vi "diSPIM Control_dual color_AB_v8.vi"(1 "Prefix for image filenames":string="A549-R11AGFP-RFP-RSV-mock-7", 3 "File Path to save DCIMG files":path=path "E:/DATA/20180315/mock") -> ()   [LabVIEW 2016]
uses:
  <userlib>/Lumenera/NiLuApi.lvlibp/Controls/LuProp.ctl
  <vilib>/DAQmx/write.llb/DAQmx Write (Analog 1D Wfm NChan NSamp).vi
  <vilib>/DAQmx/create/channels.llb/DAQmx Create Channel (AO-Voltage-Basic).vi
  <vilib>/DAQmx/configure/timing.llb/DAQmx Timing (Use Waveform).vi
  <vilib>/DAQmx/miscellaneous.llb/DAQmx Fill In Error Info.vi
  <vilib>/Instr/_visa.llb/VISA Configure Serial Port (Instr).vi
  <vilib>/ErrorRing/Error Ring.xnode
  <resource>/objmgr/daqmx.rc
  <vilib>/measure/NI_MABase.lvlib
  <userlib>/Lumenera/NiLuApi.lvlibp
  <vilib>/vision/NI_Vision_Development_Module.lvlib
panel:
  in  "Control Mode:":T1(ring) caption="Enum"
  in  "Tab Control":T2(tab)
  in  "Tab Control 4":T3(tab)=enum."SPIM Head Control"
  in  "Piezo Conversion Factor (V)":dbl=0.066
  in  "Z-Galvo Conversion \nFactor B (V)":dbl=0.0065
  in  "Z-Galvo Conversion \nFactor A (V)":dbl=0.0066
  in  "Imaging Piezo Offset (V)\n(SPIM ARM B)":dbl=5.149 min=0.0 max=10.0 step=0.001 format="%_4g"
  in  "Y-Galvo Offset B (V)":dbl=2.5 min=0.0 max=5.0 step=0.001
  in  "Imaging Piezo Offset (V)\n(SPIM ARM A)":dbl=5.487000000000003 min=0.0 max=10.0 step=0.001 format="%_4g"
  in  "Y-Galvo Offset A (V)":dbl=2.5 min=0.0 max=5.0 step=0.001
  in  "Z-Galvo Offset B (V)":dbl=2.5139999999999985 min=0.0 max=5.0 step=0.001 format="%_4g"
  in  "Z-Galvo Offset A (V)":dbl=2.5239999999999894 min=0.0 max=5.0 step=0.001 format="%_4g"
  in  "lower by":dbl=1.0 caption="um"
  in  "raise by":dbl=25000.0 caption="um"
  in  "Lower head  to 1 mm":bool caption="Lower SPIM head to find cells"
  in  "Raise head to 25 mm":bool
  in  "Lower button":bool=TRUE
  in  "Raise button":bool
  in  "Halt":bool=TRUE
  in  "Tab Control 3":T4(tab)
  out "Camera 2 Details":T5={"Model"="C11440-22C", "Camera ID"="S/N: 100720", "Firmware"="4.00.A"}
  in  "Stop SPIM \nlive":bool
  out "Camera 1 Details":T5={"Model"="C11440-22C", "Camera ID"="S/N: 100719", "Firmware"="4.00.A"}
  in  "Laser beam reference":u16(ring) items=["Right Camera", "Left Camera"]
  in  "Start SPIM \nlive":bool
  in  "Imaging":bool
  in  "Epi":bool caption="beam"
  in  "Epi scanning":bool=TRUE caption="scan"
  in  "Imaging \nscanning":bool=TRUE
  in  "BottomCam \nStop button":bool
  in  "BottomCam\n Live button":bool=TRUE
  in  "Gain":sgl(slide)=13.93722 min=0 max=14 step=0.5 scale=0.0..14.0
  in  "Exposure time (ms)":sgl(slide)=223.31839 caption="ms" min=0 max=300 step=20 scale=0.0..300.0
  in  "Raise obj \nbool":bool
  in  "Lower obj \nbool":bool
  in  "Raise obj by":dbl=10.0 caption="um"
  in  "Lower obj by":dbl=10.0 caption="um"
  in  "Tab Control 2":enum32{"Cofus alignment", "Overlay parameters"}(tab)=enum."Overlay parameters"
  in  "Z-galvo Offset A slider":dbl(slide) scale=-30.0..30.0
  in  "Z-galvo Offset B slider":dbl(slide)=0.15873015873015817 scale=-30.0..30.0
  in  "Overlay Color":u32(colorbox)
  in  "Choose Overlay":u16(ring)=2 items=["No overlay", "x", "+"]
  in  "lower threshold":u16(slide)=88 scale=0.0..150.0
  in  "higher threshold":u16(slide)=20000 min=124 scale=100.0..20000.0
  in  "mid-level":u16(slide)=1709 min=124 max=50994 scale=100.0..6000.0
  out "Right spim Camera image":T6(plugin-control) caption="Right SPIM Cam"
  in  "Stop Adjustment":bool
  out "Waveform Graph":sgl[](graph)=[101.0, 104.0, 103.0, 99.0, 104.0, 97.0, 103.0, 98.0, 108.0, 97.0, 100.0, 98.0, 98.0, 99.0, 99.0, 105.0, 101.0, 103.0, 101.0, 106.0, 101.0, 104.0, 101.0, 104.0, 106.0, 87.0, 96.0, 98.0, 100.0, 99.0, 100.0, 99.0, 106.0, 103.0, 104.0, 103.0, 110.0, 104.0, 98.0, 101.0, 105.0, 100.0, 94.0, 103.0, 101.0, 105.0, 103.0, 107.0, 104.0, 103.0, 96.0, 110.0, 104.0, 99.0, 109.0, 101.0, 97.0, 98.0, 101.0, 101.0, 102.0, 107.0, 98.0, 106.0, 105.0, 108.0, 91.0, 106.0, 100.0, 101.0, 104.0, 101.0, 121.0, 105.0, 107.0, 101.0, 107.0, 101.0, 85.0, 104.0, 100.0, 104.0, 105.0, 107.0, 101.0, 103.0, 101.0, 101.0, 96.0, 107.0, 100.0, 98.0, 104.0, 101.0, 100.0, 105.0, 108.0, 104.0, 90.0, 104.0, 105.0, 103.0, 109.0, 108.0, 98.0, 105.0, 105.0, 108.0, 100.0, 109.0, 103.0, 104.0, 107.0, 103.0, 98.0, 99.0, 106.0, 106.0, 99.0, 107.0, 99.0, 100.0, 102.0, 101.0, 108.0, 98.0, 98.0, 105.0, 100.0, 100.0, 107.0, 107.0, 98.0, 106.0, 104.0, 102.0, 116.0, 108.0, 104.0, 100.0, 99.0, 100.0, 101.0, 100.0, 103.0, 108.0, 102.0, 113.0, 108.0, 110.0, 122.0, 108.0, 101.0, 110.0, 105.0, 108.0, 101.0, 107.0, 109.0, 108.0, 104.0, 114.0, 107.0, 108.0, 111.0, 102.0, 118.0, 107.0, 117.0, 117.0, 103.0, 101.0, 105.0, 110.0, 105.0, 112.0, 112.0, 115.0, 106.0, 119.0, 105.0, 115.0, 113.0, 121.0, 110.0, 108.0, 110.0, 115.0, 112.0, 113.0, 112.0, 108.0, 115.0, 109.0, 102.0, 115.0, 112.0, 113.0, 115.0, 126.0, 125.0, 105.0, 120.0, 116.0, 125.0, 122.0, 115.0, 107.0, 111.0, 136.0, 115.0, 123.0, 116.0, 126.0, 115.0, 123.0, 132.0, 142.0, 129.0, 146.0, 134.0, 145.0, 140.0, 152.0, 143.0, 148.0, 143.0, 140.0, 170.0, 170.0, 202.0, 208.0, 209.0, 234.0, 232.0, 276.0, 293.0, 298.0, 361.0, 427.0, 415.0, 450.0, 477.0, 544.0, 541.0, 653.0, 643.0, 756.0, 771.0, 801.0, 810.0, 930.0, 954.0, 970.0, 1079.0, 1072.0, 1191.0, 1148.0, 1110.0, 1097.0, 1055.0, 942.0, 881.0, 839.0, 731.0, 669.0, 626.0, 534.0, 535.0, 474.0, 363.0, 352.0, 342.0, 280.0, 315.0, 253.0, 270.0, 247.0, 229.0, 206.0, 203.0, 187.0, 158.0, 163.0, 175.0, 145.0, 154.0, 158.0, 147.0, 138.0, 121.0, 130.0, 126.0, 120.0, 131.0, 121.0, 119.0, 113.0, 120.0, 125.0, 113.0, 122.0, 130.0, 129.0, 114.0, 115.0, 106.0, 127.0, 124.0, 112.0, 120.0, 105.0, 117.0, 115.0, 125.0, 110.0, 111.0, 113.0, 124.0, 106.0, 117.0, 117.0, 119.0, 127.0, 131.0, 118.0, 124.0, 128.0, 121.0, 116.0, 108.0, 107.0, 102.0, 115.0, 112.0, 124.0, 112.0, 124.0, 108.0, 118.0, 105.0, 119.0, 109.0, 111.0, 109.0, 119.0, 108.0, 111.0, 107.0, 117.0, 111.0, 104.0, 106.0, 114.0, 110.0, 115.0, 113.0, 105.0, 118.0, 116.0, 110.0, 104.0, 106.0, 120.0, 101.0, 104.0, 102.0, 110.0, 99.0, 112.0, 112.0, 99.0, 110.0, 109.0, 115.0, 104.0, 107.0, 104.0, 108.0, 102.0, 106.0, 112.0, 106.0, 108.0, 104.0, 110.0, 108.0, 104.0, 106.0, 106.0, 96.0, 113.0, 108.0, 99.0, 112.0, 110.0, 109.0, 112.0, 107.0, 94.0, 108.0, 103.0, 106.0, 108.0, 108.0, 101.0, 113.0, 101.0, 100.0, 101.0, 107.0, 93.0, 104.0, 100.0, 100.0, 103.0, 101.0, 108.0, 113.0, 108.0, 89.0, 107.0, 105.0, 109.0, 106.0, 103.0, 106.0, 117.0, 100.0, 108.0, 103.0, 105.0, 104.0, 101.0, 100.0, 105.0, 109.0, 108.0, 105.0, 109.0, 106.0, 104.0, 98.0, 102.0, 98.0, 104.0, 107.0, 100.0, 106.0, 102.0, 101.0, 99.0, 106.0, 109.0, 101.0, 105.0, 106.0, 116.0, 101.0, 104.0, 105.0, 102.0, 106.0, 103.0, 100.0, 101.0, 101.0, 105.0, 103.0, 105.0, 108.0, 109.0, 97.0, 108.0, 105.0, 99.0, 110.0, 110.0, 108.0, 102.0, 100.0, 103.0, 109.0, 111.0, 104.0, 106.0, 108.0, 105.0, 101.0, 98.0, 100.0, 98.0, 101.0, 98.0, 101.0, 107.0, 100.0, 101.0, 101.0, 103.0, 101.0, 106.0, 101.0, 101.0, 104.0, 112.0, 101.0, 99.0, 105.0, 104.0, 100.0, 110.0]
  out "Left spim Camera image":T6(plugin-control) caption="Left SPIM Cam"
  in  "LED power":i32(slide) min=0 max=100 step=1 scale=0.0..100.0
  in  "Switch to internal":bool
  out "Scanner/Piezo \ncontrol mode":string="Already in external (NI-DAQ)"
  out "Waveform Graph 2":sgl[](graph)=[102.0, 99.0, 106.0, 109.0, 108.0, 102.0, 107.0, 106.0, 103.0, 111.0, 105.0, 99.0, 105.0, 102.0, 104.0, 102.0, 103.0, 104.0, 107.0, 107.0, 104.0, 110.0, 105.0, 106.0, 109.0, 101.0, 109.0, 101.0, 103.0, 105.0, 103.0, 101.0, 100.0, 106.0, 106.0, 100.0, 101.0, 101.0, 107.0, 101.0, 104.0, 103.0, 101.0, 111.0, 102.0, 107.0, 100.0, 104.0, 109.0, 108.0, 107.0, 101.0, 108.0, 103.0, 105.0, 102.0, 107.0, 107.0, 100.0, 98.0, 104.0, 114.0, 98.0, 106.0, 102.0, 115.0, 109.0, 111.0, 102.0, 99.0, 110.0, 116.0, 101.0, 107.0, 104.0, 106.0, 112.0, 104.0, 106.0, 95.0, 104.0, 103.0, 110.0, 107.0, 104.0, 105.0, 102.0, 110.0, 101.0, 107.0, 104.0, 111.0, 100.0, 102.0, 115.0, 111.0, 118.0, 99.0, 108.0, 100.0, 100.0, 105.0, 107.0, 105.0, 117.0, 101.0, 114.0, 112.0, 102.0, 111.0, 103.0, 113.0, 106.0, 107.0, 110.0, 105.0, 108.0, 111.0, 101.0, 108.0, 113.0, 111.0, 103.0, 112.0, 105.0, 101.0, 117.0, 111.0, 105.0, 107.0, 105.0, 114.0, 113.0, 98.0, 102.0, 115.0, 114.0, 107.0, 105.0, 113.0, 114.0, 114.0, 119.0, 111.0, 100.0, 114.0, 114.0, 106.0, 110.0, 115.0, 111.0, 108.0, 124.0, 112.0, 105.0, 123.0, 111.0, 109.0, 117.0, 111.0, 110.0, 118.0, 109.0, 111.0, 103.0, 113.0, 113.0, 111.0, 104.0, 108.0, 106.0, 123.0, 114.0, 108.0, 119.0, 118.0, 120.0, 126.0, 124.0, 108.0, 121.0, 123.0, 111.0, 122.0, 121.0, 117.0, 115.0, 126.0, 113.0, 127.0, 139.0, 125.0, 122.0, 126.0, 132.0, 162.0, 146.0, 141.0, 142.0, 130.0, 159.0, 159.0, 198.0, 172.0, 207.0, 211.0, 256.0, 274.0, 308.0, 402.0, 428.0, 376.0, 428.0, 645.0, 602.0, 716.0, 602.0, 661.0, 566.0, 594.0, 553.0, 512.0, 490.0, 361.0, 363.0, 257.0, 258.0, 264.0, 251.0, 258.0, 256.0, 262.0, 248.0, 299.0, 221.0, 221.0, 170.0, 167.0, 172.0, 150.0, 143.0, 153.0, 142.0, 156.0, 155.0, 118.0, 159.0, 150.0, 143.0, 154.0, 134.0, 144.0, 152.0, 151.0, 161.0, 169.0, 163.0, 147.0, 179.0, 176.0, 174.0, 161.0, 175.0, 217.0, 228.0, 253.0, 288.0, 374.0, 510.0, 661.0, 735.0, 851.0, 1145.0, 1247.0, 1085.0, 773.0, 617.0, 484.0, 393.0, 392.0, 316.0, 287.0, 216.0, 197.0, 195.0, 173.0, 170.0, 159.0, 147.0, 152.0, 124.0, 131.0, 116.0, 119.0, 107.0, 107.0, 113.0, 104.0, 113.0, 114.0, 108.0, 114.0, 103.0, 107.0, 105.0, 111.0, 104.0, 100.0, 101.0, 104.0, 105.0, 97.0, 98.0, 95.0, 111.0, 101.0, 108.0, 105.0, 103.0, 107.0, 114.0, 103.0, 109.0, 106.0, 107.0, 93.0, 99.0, 101.0, 104.0, 103.0, 101.0, 107.0, 100.0, 96.0, 99.0, 100.0, 104.0, 106.0, 101.0, 110.0, 108.0, 102.0, 100.0, 101.0, 105.0, 98.0, 102.0, 103.0, 101.0, 97.0, 105.0, 104.0, 102.0, 100.0, 101.0, 105.0, 100.0, 107.0, 101.0, 105.0, 101.0, 100.0, 102.0, 99.0, 103.0, 111.0, 103.0, 105.0, 102.0, 100.0, 108.0, 98.0, 101.0, 105.0, 97.0, 101.0, 100.0, 101.0, 103.0, 109.0, 103.0, 101.0, 100.0, 105.0, 99.0, 102.0, 103.0, 97.0, 107.0, 105.0, 101.0, 100.0, 101.0, 101.0, 103.0, 101.0, 101.0, 105.0, 104.0, 101.0, 96.0, 101.0, 97.0, 102.0, 103.0, 102.0, 101.0, 111.0, 103.0, 102.0, 101.0, 106.0, 100.0, 108.0, 101.0, 103.0, 102.0, 102.0, 103.0, 104.0, 100.0, 109.0, 105.0, 101.0, 100.0, 99.0, 102.0, 95.0, 98.0, 107.0, 98.0, 103.0, 104.0, 101.0, 101.0, 106.0, 101.0, 102.0, 103.0, 99.0, 103.0, 99.0, 97.0, 99.0, 100.0, 101.0, 111.0, 102.0, 100.0, 104.0, 98.0, 100.0, 118.0, 100.0, 100.0, 105.0, 100.0, 99.0, 103.0, 117.0, 101.0, 104.0, 102.0, 101.0, 100.0, 102.0, 101.0, 102.0, 100.0, 102.0, 100.0, 103.0, 99.0, 100.0, 106.0, 103.0, 102.0, 104.0, 105.0, 103.0, 99.0, 103.0, 102.0, 100.0, 99.0, 94.0, 101.0, 102.0, 101.0, 100.0, 101.0, 104.0, 106.0, 99.0, 106.0, 95.0, 100.0, 102.0, 102.0, 101.0, 101.0, 100.0, 101.0, 105.0, 95.0, 88.0, 98.0, 98.0, 100.0, 98.0, 98.0, 108.0]
  in  "Bgndbool":bool=TRUE
  in  "Autofocus \n(move only galvo )":bool
  in  "Time/Plane":dbl=5.0 caption="ms"
  in  "Z Step Size":dbl=0.5 caption="um" min=0.0 max=2.0
  in  "# Planes/Volume":dbl=50.0
  in  "# of Volumes":dbl=500.0
  in  "Time Point Delay":dbl caption="ms"
  in  "Laser power (488 nm)":dbl(slide) min=0.0 max=10.0 step=0.1 scale=0.0..10.0
  in  "Laser power (561 nm)":dbl(slide) min=0.0 max=10.0 step=0.1 scale=0.0..10.0
  in  "Light Sheet Width":dbl=40.0 caption="um"
  out "Volume Indicator":dbl(slide)=499.0 max=10.0 scale=0.0..500.0
  out "planes acquired (B)":dbl=49.0 caption="SPIM B"
  out "planes acquired (A)":dbl=49.0 caption="SPIM A"
  in  "Export to TIFF":bool
  out "Acquisition status:":string="Done."
  out "Camera A ID:":string="S/N: 100719"
  out "Camera B ID:":string="S/N: 100720"
  in  "Camera SPIMB":T7={"Horizontal Offset"=772, "Vertical Offset"=772, "Horizontal Width"=512, "Vertical Width"=512}
  in  "Camera SPIMA":T7={"Horizontal Offset"=772, "Vertical Offset"=772, "Horizontal Width"=512, "Vertical Width"=512}
  out "TIFF storage for SPIM ARM B":path=path "E:/DATA/20180315/mock/A549-R11AGFP-RFP-RSV-mock-7/ARM2"
  out "TIFF storage for SPIM ARM A":path=path "E:/DATA/20180315/mock/A549-R11AGFP-RFP-RSV-mock-7/ARM1"
  in  "AutoFocus \n(move only piezo)":bool caption="AutoFocus"
  out "SPIM Camera Error":errorcluster {"code" format="%.0x"}
  out "SPIMA DAQ Error":errorcluster
  out "SPIMB DAQ Error":errorcluster
  out "Bottom Cam error":errorcluster
  in  "X-Position":dbl
  in  "Y-Position":dbl
  in  "F-Axis Position":dbl
  in  "File Name":string
  out "DAQ1 error (adjustment)":errorcluster
  out "DAQ2 error (adjustment)":errorcluster
  out "File conversion error":errorcluster
  out "stage2":u32=267
  out "stage1":u32=268
  out "stage 3":u32=37
  out "interstage":u32=1
  out "stage0":u32=113
  out "Serial port errors":errorcluster
  in  "Capture Images On/Off":bool=TRUE
  out "stage0 2":u32=174
  out "interstage 2":u32=1
  out "stage 4":u32=54
  out "stage2 2":u32=600
  out "stage1 2":u32=547
  out "File conversion Dual color":errorcluster
  out "BottomCam\n frameRate out":sgl=20.58668
  in  "Force Cameras Open":bool
  out "Imag. cond. error out":errorcluster
  # "Galvo & Piezo Control"
  # "SPIM A"
  # "SPIM B"
  # "SPIM head motion"
  # "Scouting camera control"
  # "Storage for DCIMG image files"
  # "Image Acquisition Parameters"
  # "Imaging progress indicators"
  # "Storage for TIFF files post export"
  # "Camera Control parameters"
  # "Saving Front Panel Parameters"
  # "Single color timing"
  # "Dual color timing"
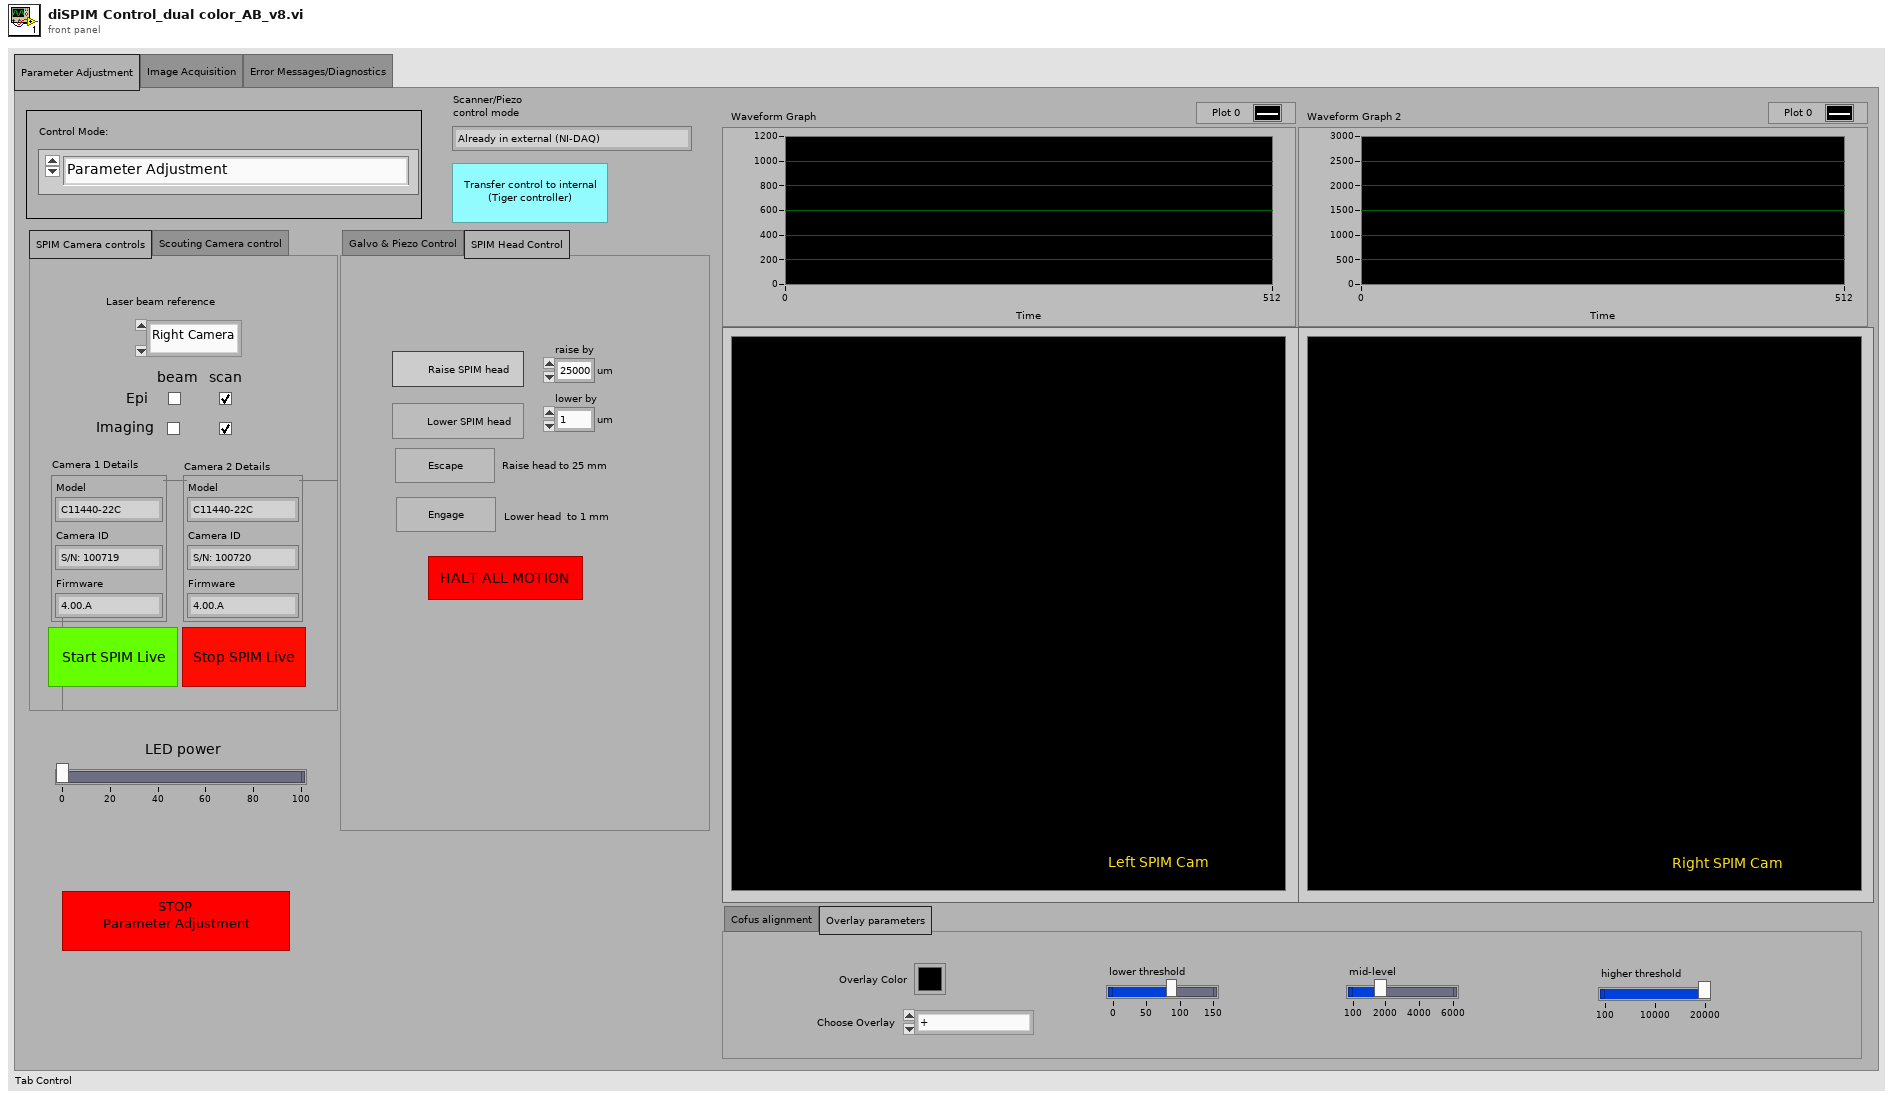
[diagram p1: front panel]
types:
  T1 = enum32{"Parameter Adjustment", "Image Acquisition - Single Color", "Image Acquisition - Dual Color"}
  T2 = enum32{"Parameter Adjustment", "Image Acquisition", "Error Messages/Diagnostics"}
  T3 = enum32{"Galvo & Piezo Control", "SPIM Head Control"}
  T4 = enum32{"SPIM Camera controls", "Scouting Camera control"}
  T5 = cluster{"Model":string, "Camera ID":string, "Firmware":string}
  T6 = typedef "IMAQ Image.ctl" = refnum<image>
  T7 = cluster{"Horizontal Offset":i32, "Vertical Offset":i32, "Horizontal Width":i32, "Vertical Width":i32}
  T8 = cluster{"cTime/plane":dbl, "cNoOfVol":dbl, "cZStepSize":dbl, "cTimePointDelay":dbl, "cPlanes/Vol":dbl, "cLightShtWdth":dbl, "cLasPow488":dbl, "cLasPow561":dbl, "cZGalOffA":dbl, "cZGalOffB":dbl, "cZGalConvFacA":dbl, "cZGalConvFacB":dbl, "cYGalOffA":dbl, "cYGalOffB":dbl, "cPzOffB":dbl, "cPzOffA":dbl, "cPzConvFac":dbl}
  T9 = cluster{"Y-Gal ampl":dbl, "A Z-Gal amp":dbl, "A Z-Gal Off":dbl, "Imag Obj Amp":dbl, "A Obj Off H":dbl, "A Obj Off L":dbl, "B Obj Off H":dbl, "B Obj Off L":dbl, "B Z-Gal Amp":dbl, "B Z-Gal Off":dbl, "488 laser pow":dbl, "561 laser pow":dbl, "A Y-Gal Off":dbl, "B Y-Gal Off ":dbl, "planes/vol":dbl, "Time/plane":dbl}
  T10 = cluster{"Demosaicing Method":u32, "Correction Matrix":u32}
  T11 = enum16{"Sine Wave", "Triangle Wave", "Square Wave", "Sawtooth Wave"}
  T12 = cluster{"height":u32, "width":u32, "datatype":u32}
  T13 = typedef "Image Type" = u32
  T14 = typedef "NiLuApi.lvlibp/LuProp.ctl" = u32
  T15 = cluster{"Size":u32, "Width":u32, "Height":u32, "Pixel Format":u32, "Image Size":u32, "Reserve 1":u32, "Reserve 2":u32, "Reserve 3":u32, "Reserve 4":u32, "Reserve 5":u32, "Reserve 6":u32, "Reserve 7":u32, "Reserve 8":u32}
  T16 = typedef "NiLuApi.lvlibp/IMAQ Image.ctl" = refnum<image>
  T17 = cluster{"DAQ1":waveform(dbl)[], "DAQ 2":waveform(dbl)[]}
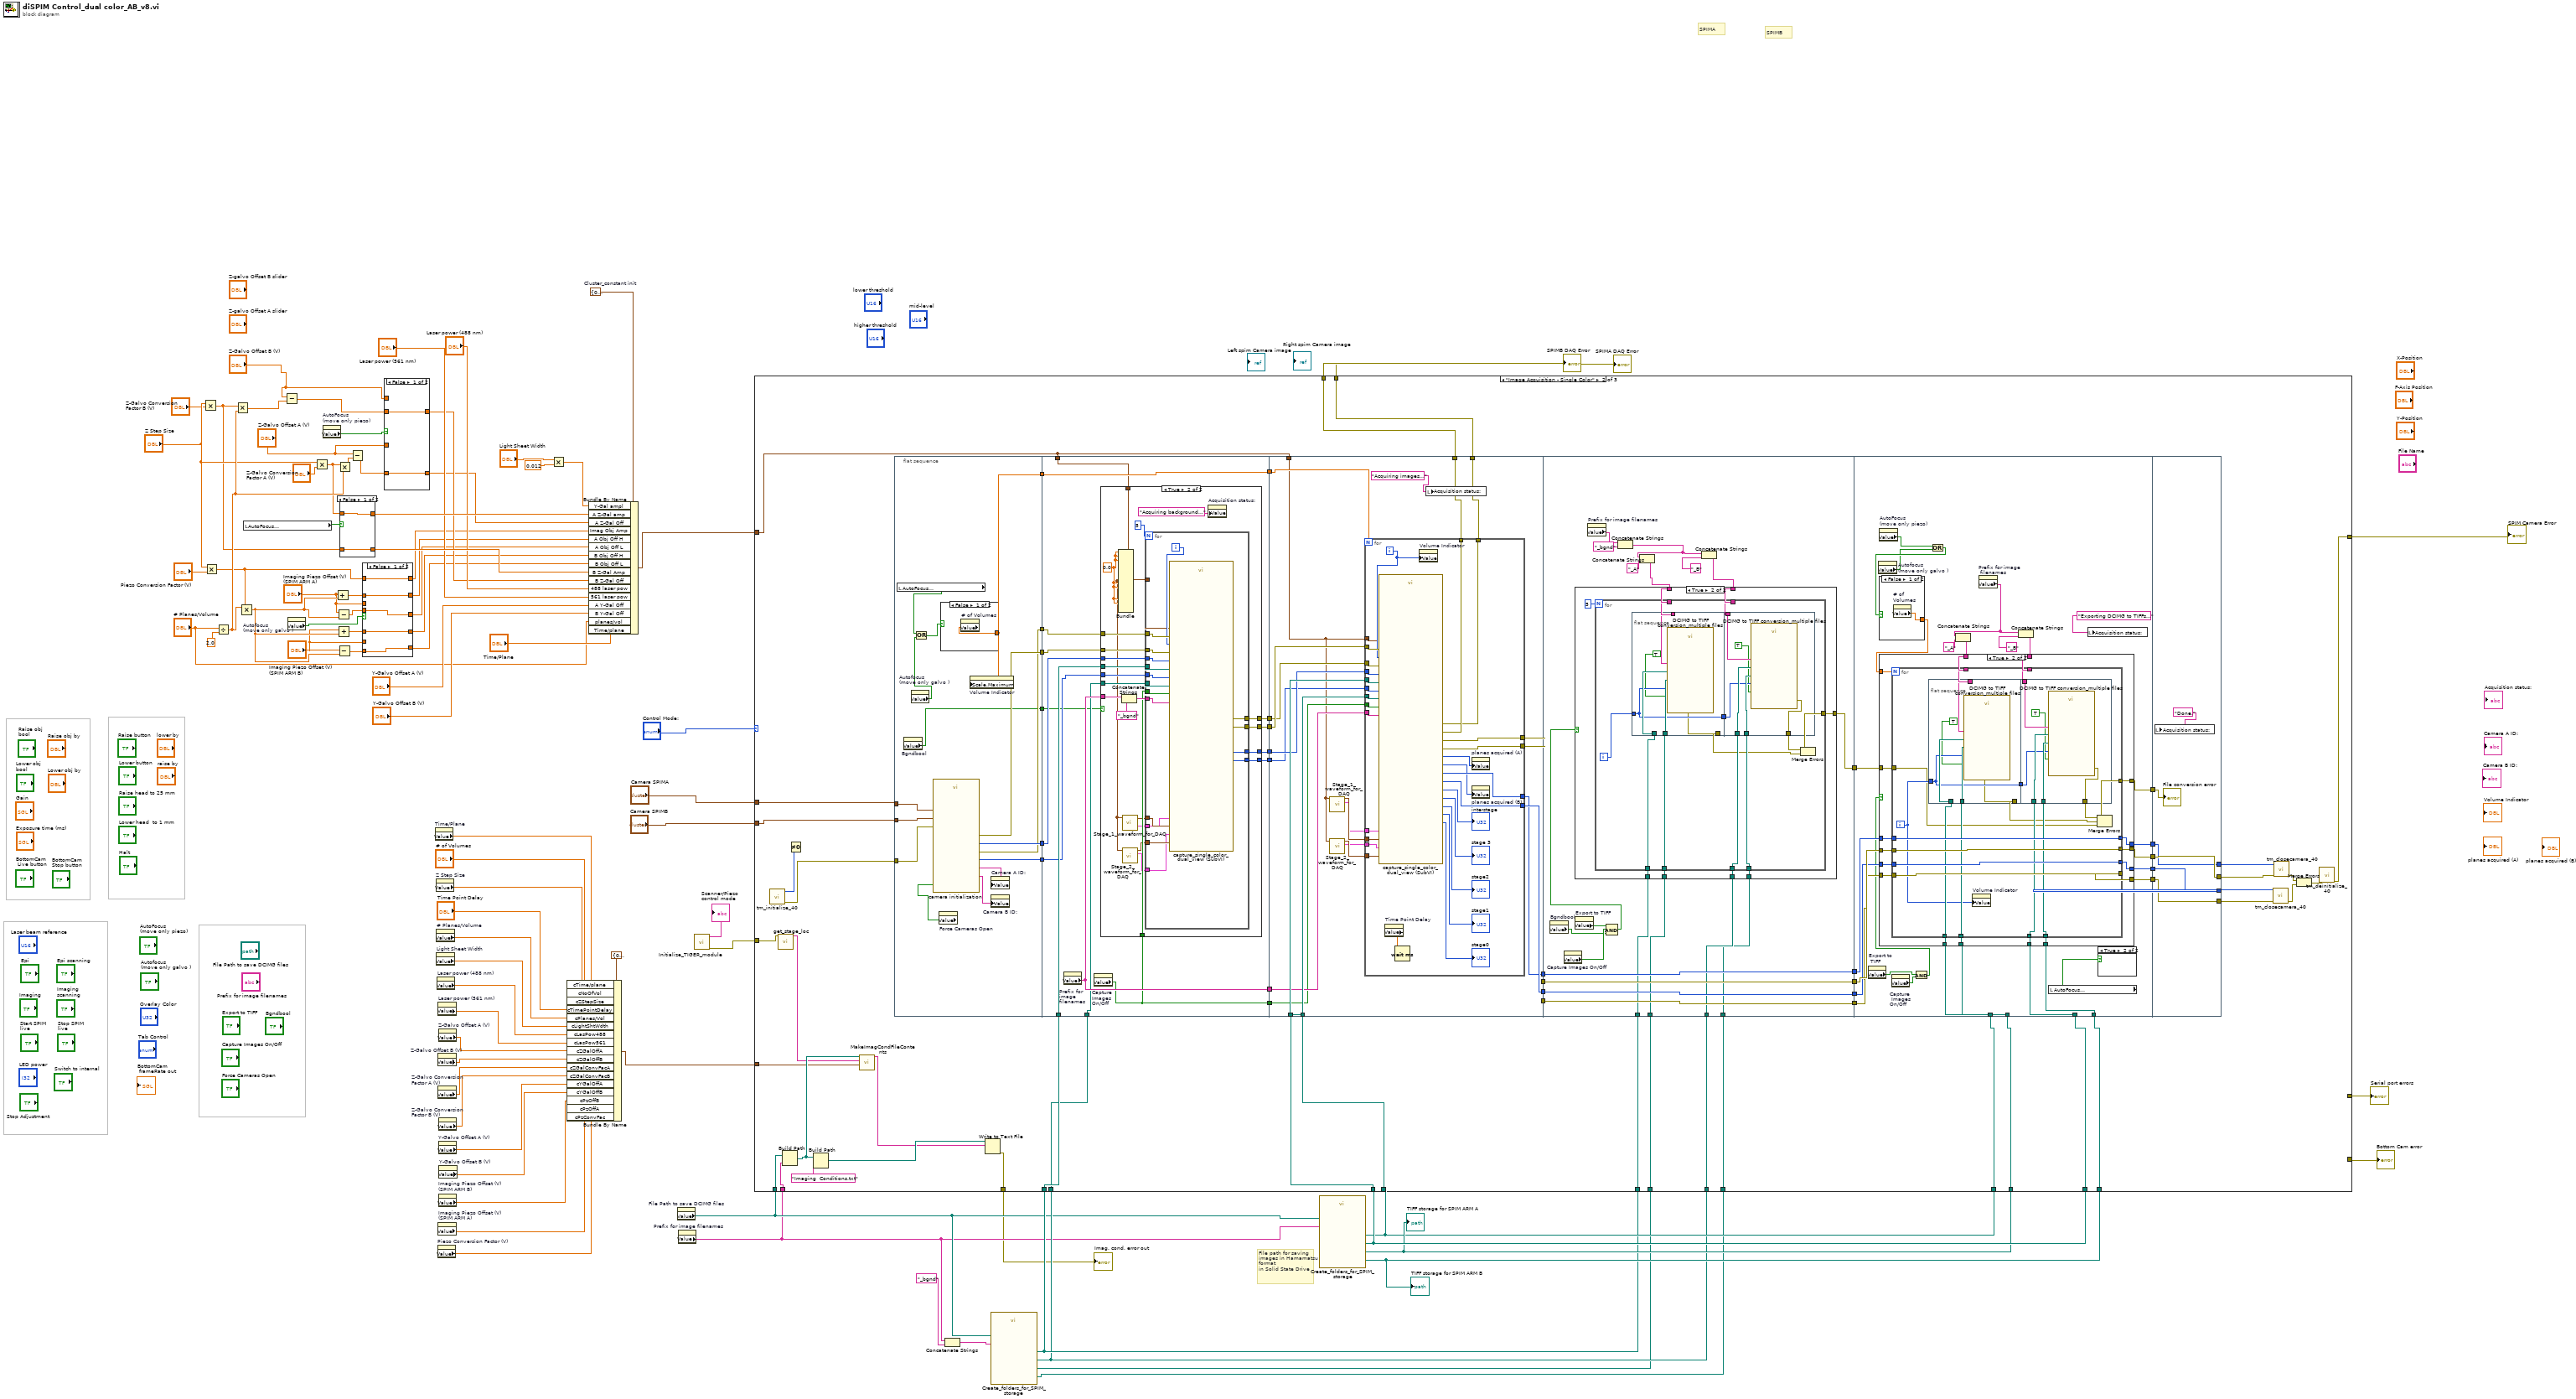
[diagram p0: block diagram]
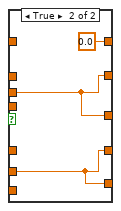
[diagram p2: hidden frame]
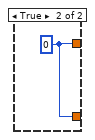
[diagram p4: hidden frame]
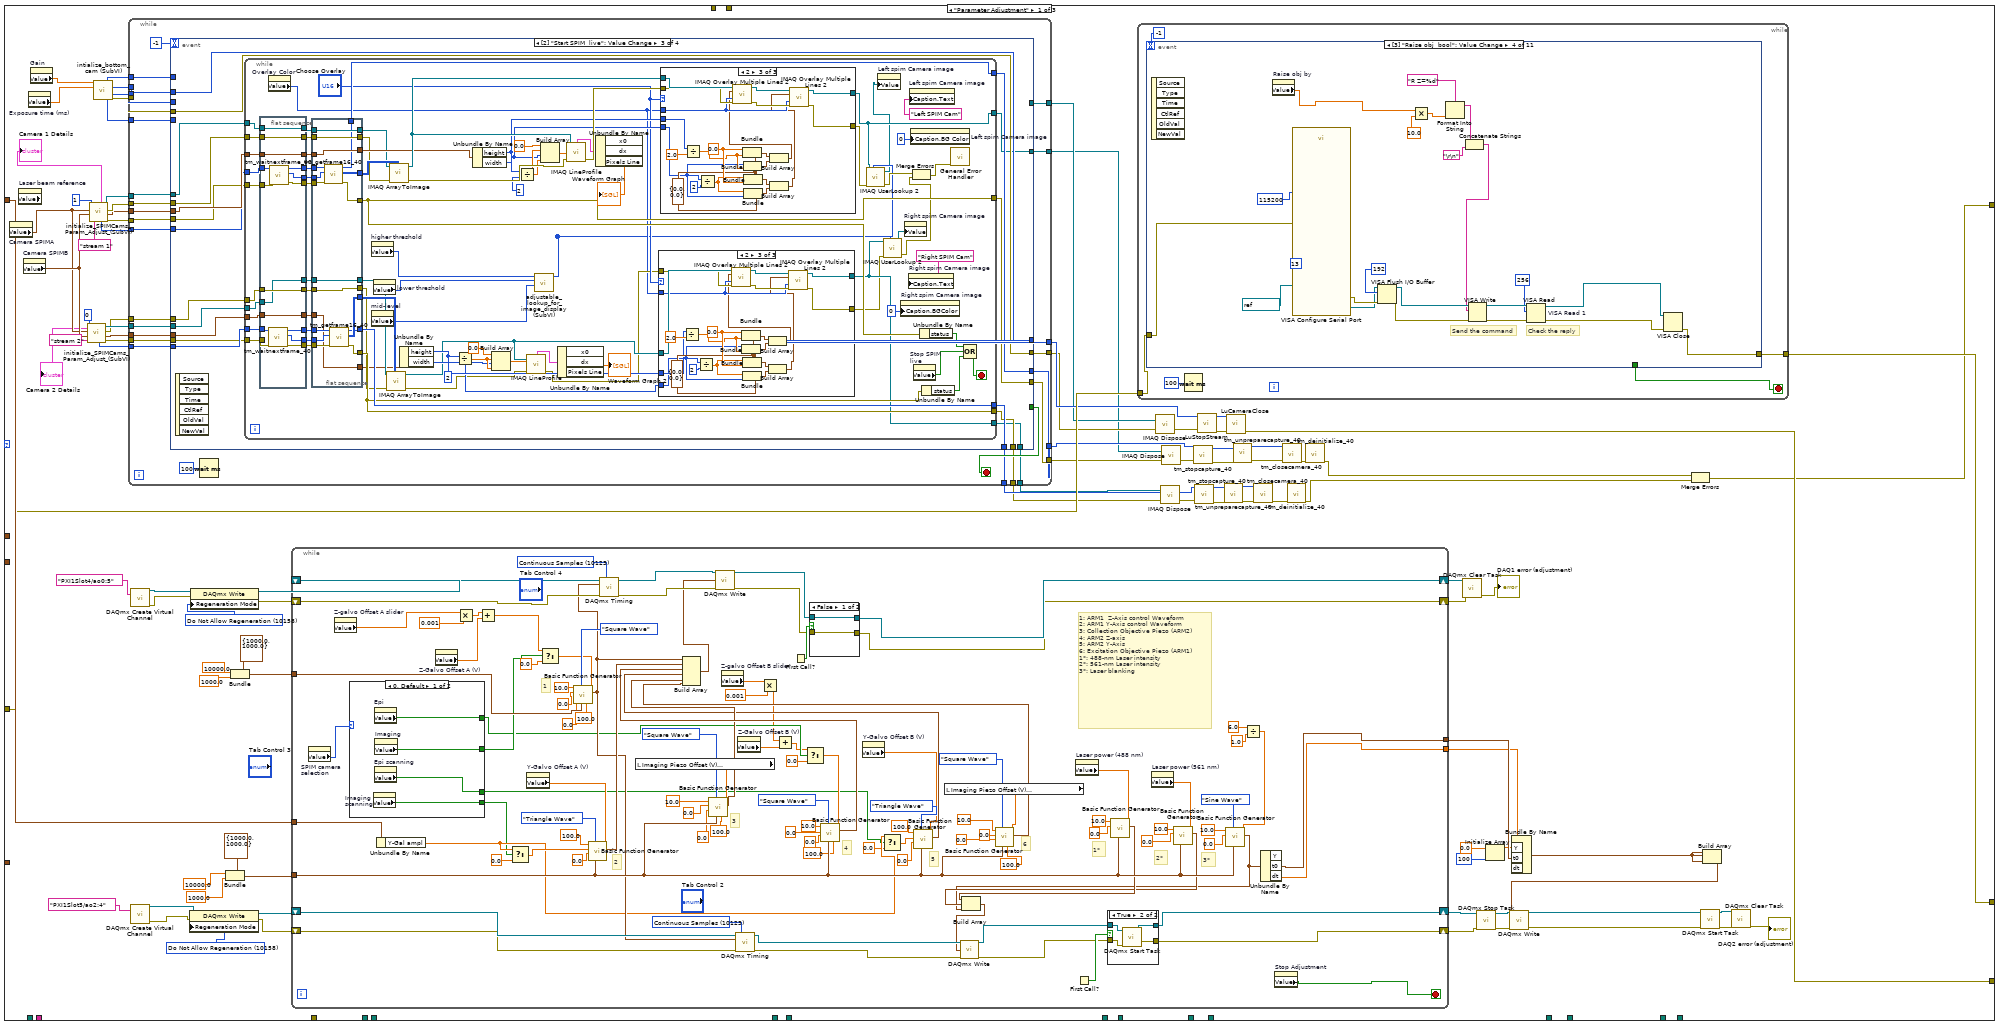
[diagram p5: hidden frame]
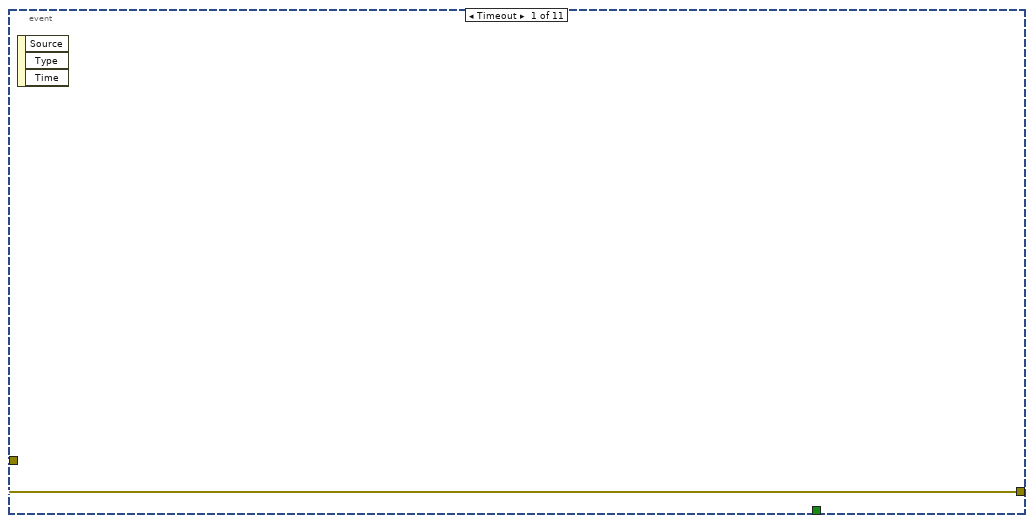
[diagram p6: hidden frame]
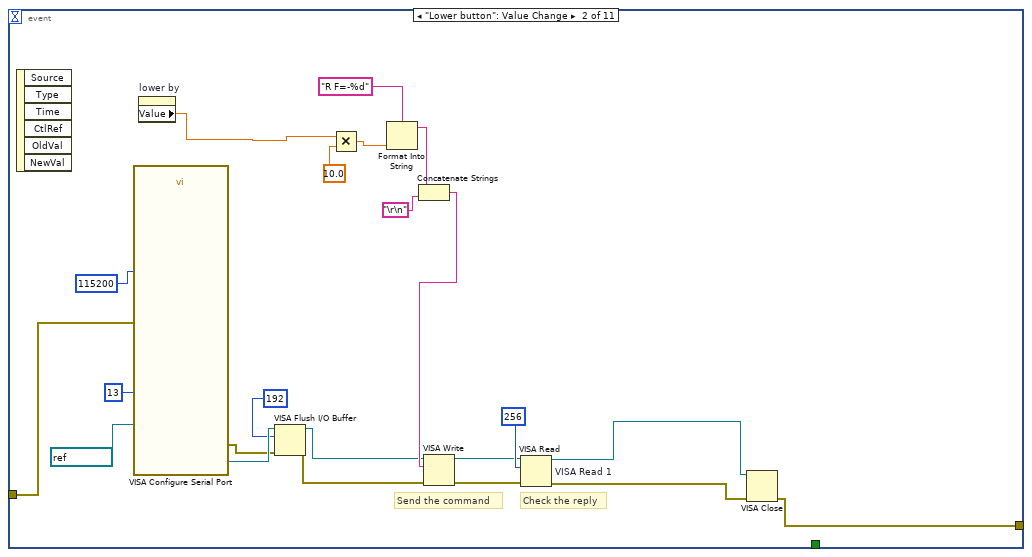
[diagram p7: hidden frame]
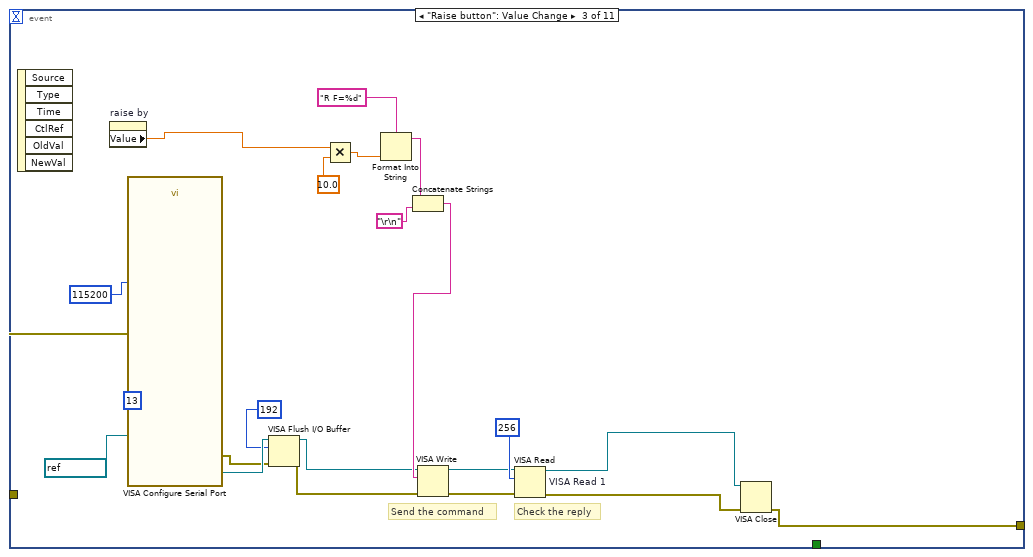
[diagram p8: hidden frame]
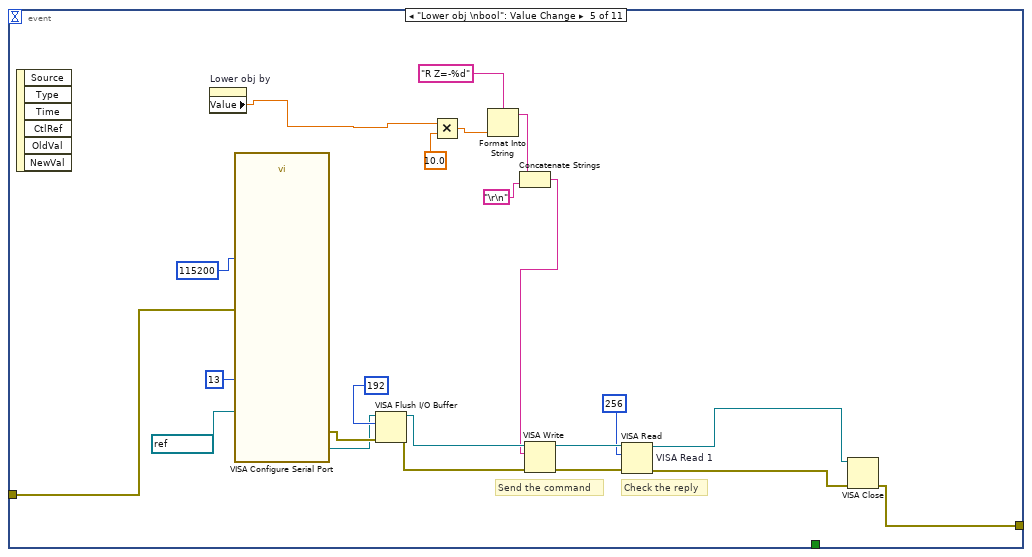
[diagram p9: hidden frame]
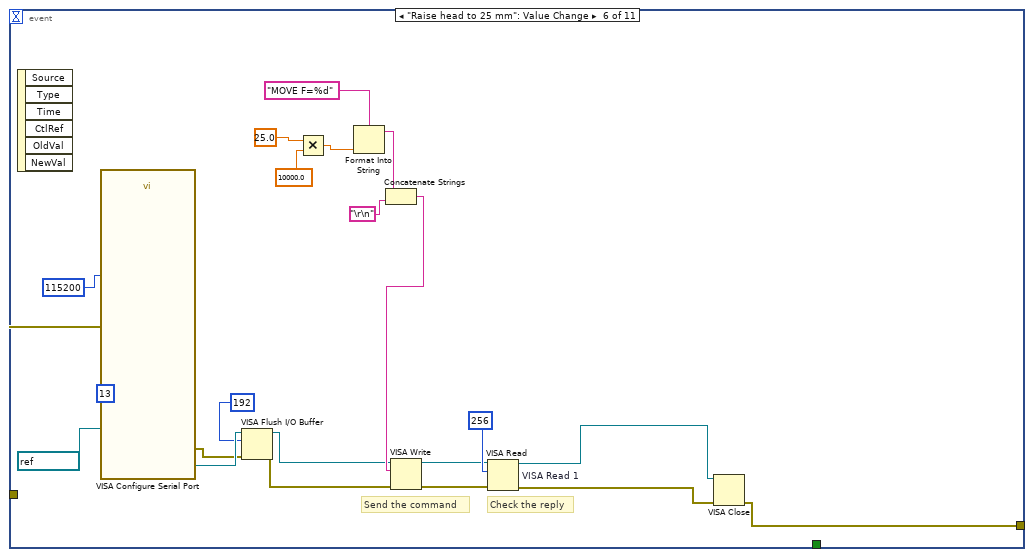
[diagram p10: hidden frame]
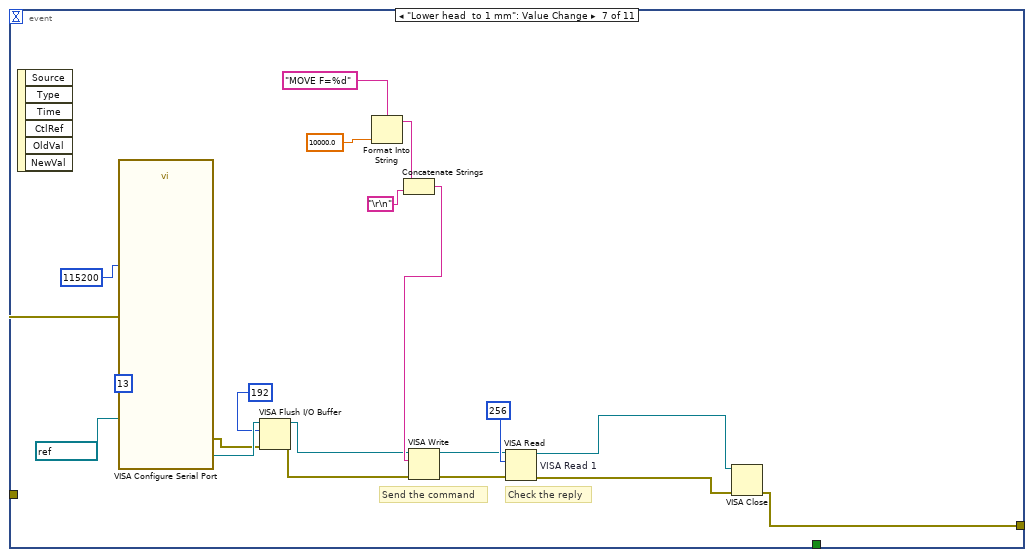
[diagram p11: hidden frame]
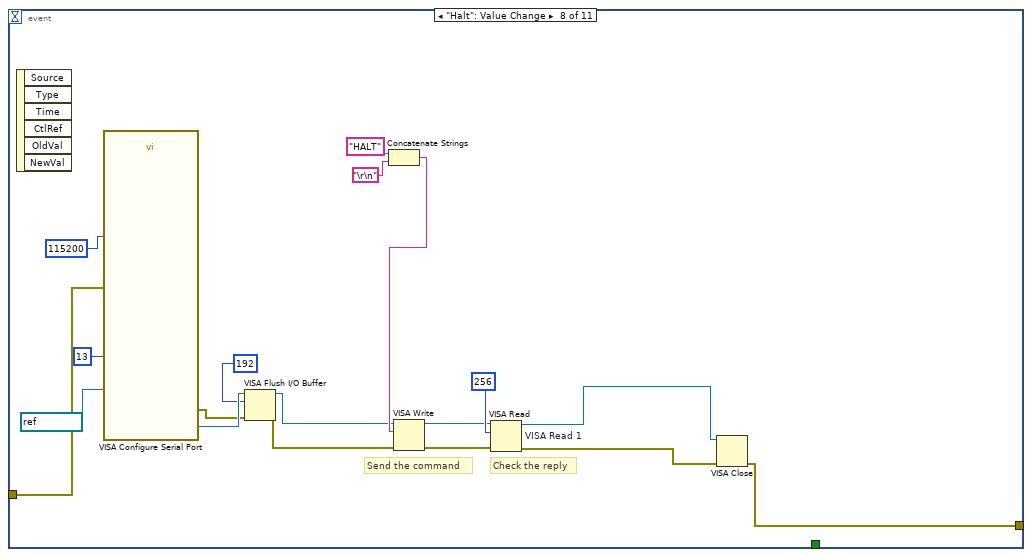
[diagram p12: hidden frame]
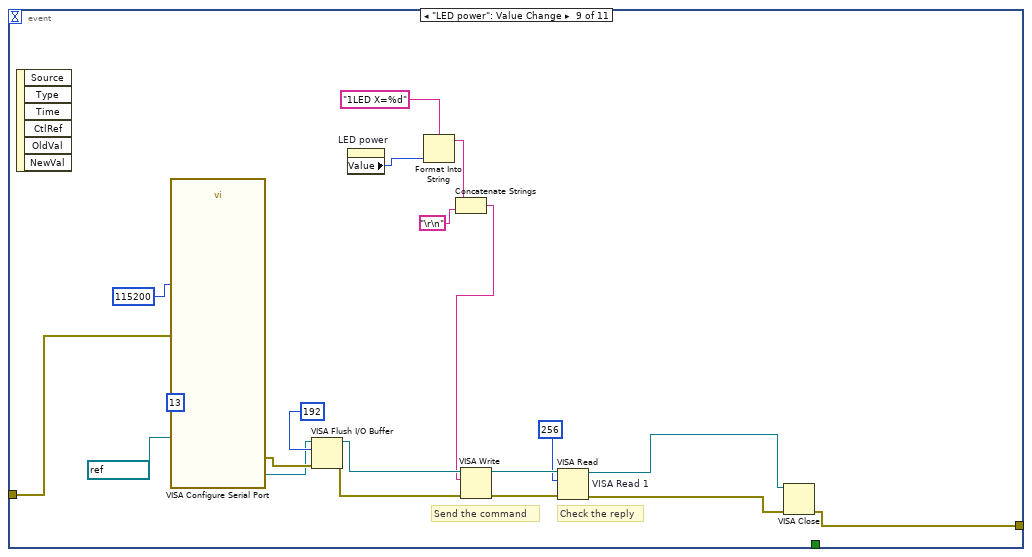
[diagram p13: hidden frame]
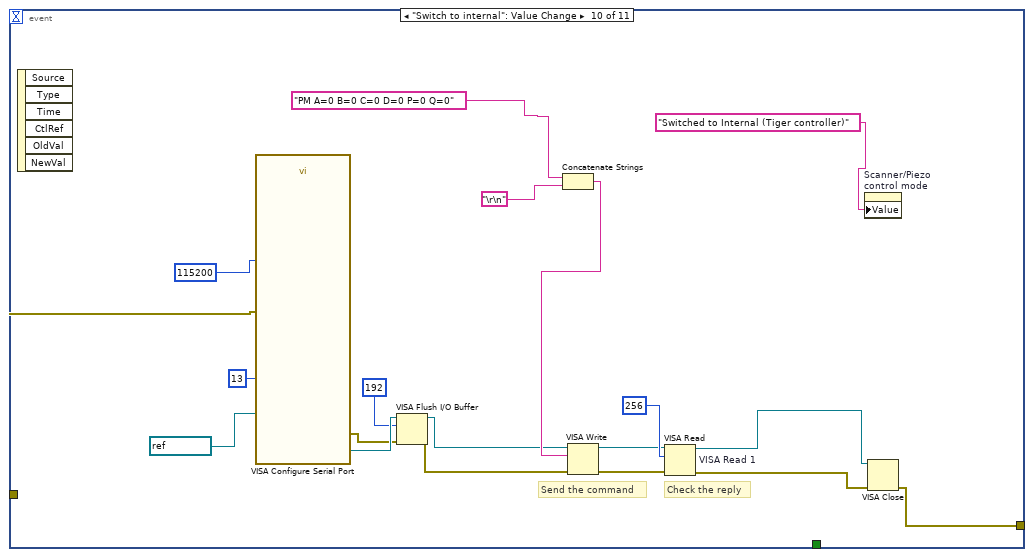
[diagram p14: hidden frame]
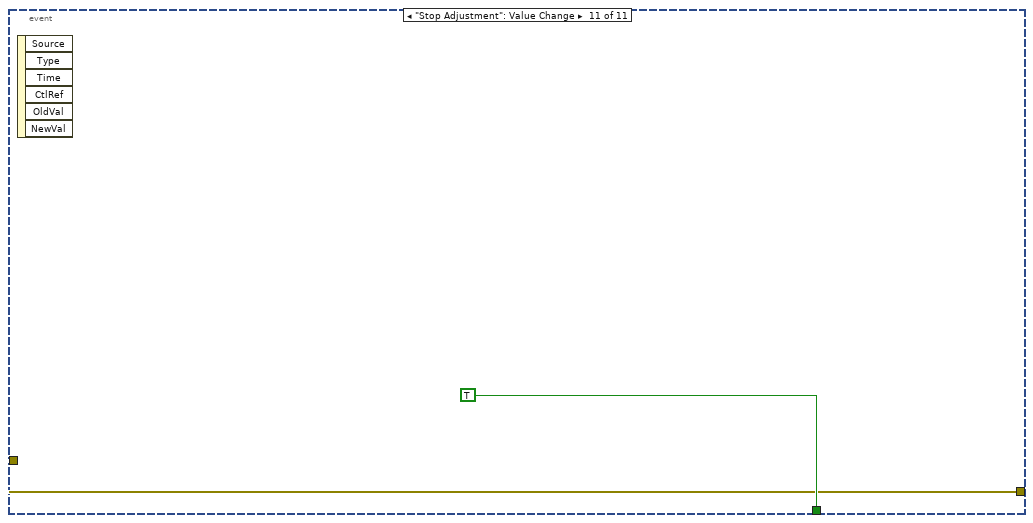
[diagram p15: hidden frame]
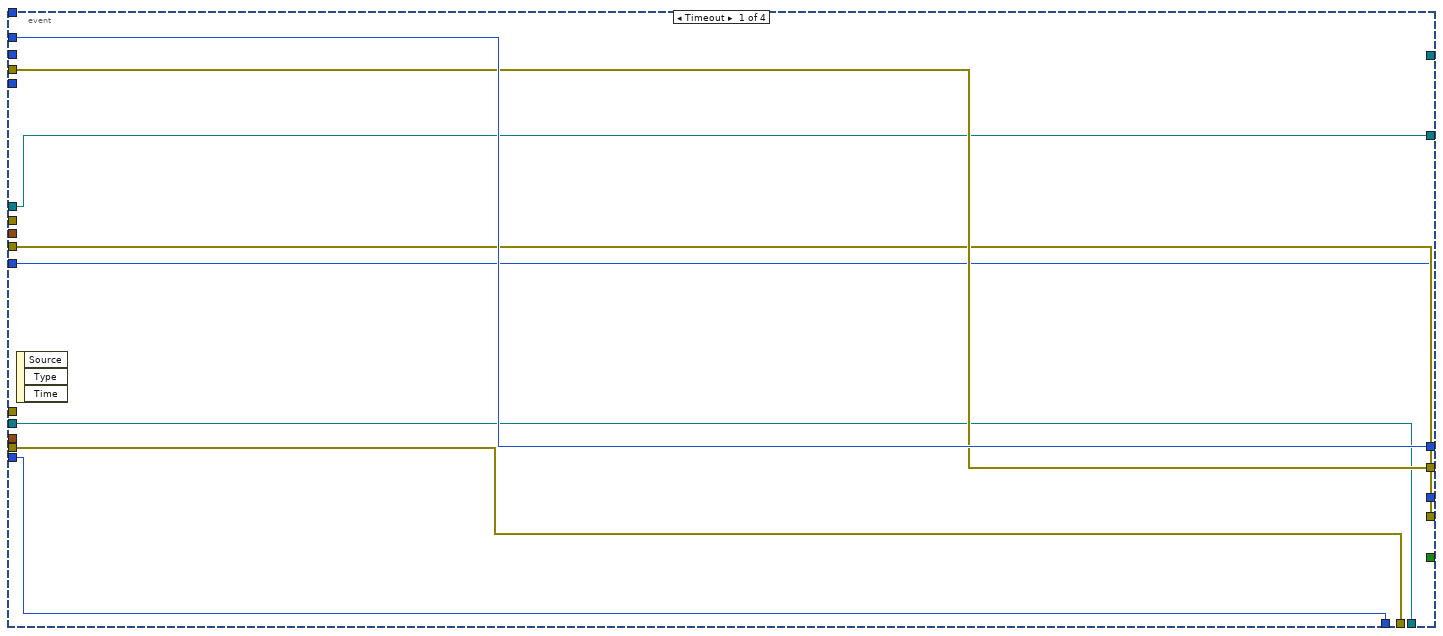
[diagram p16: hidden frame]
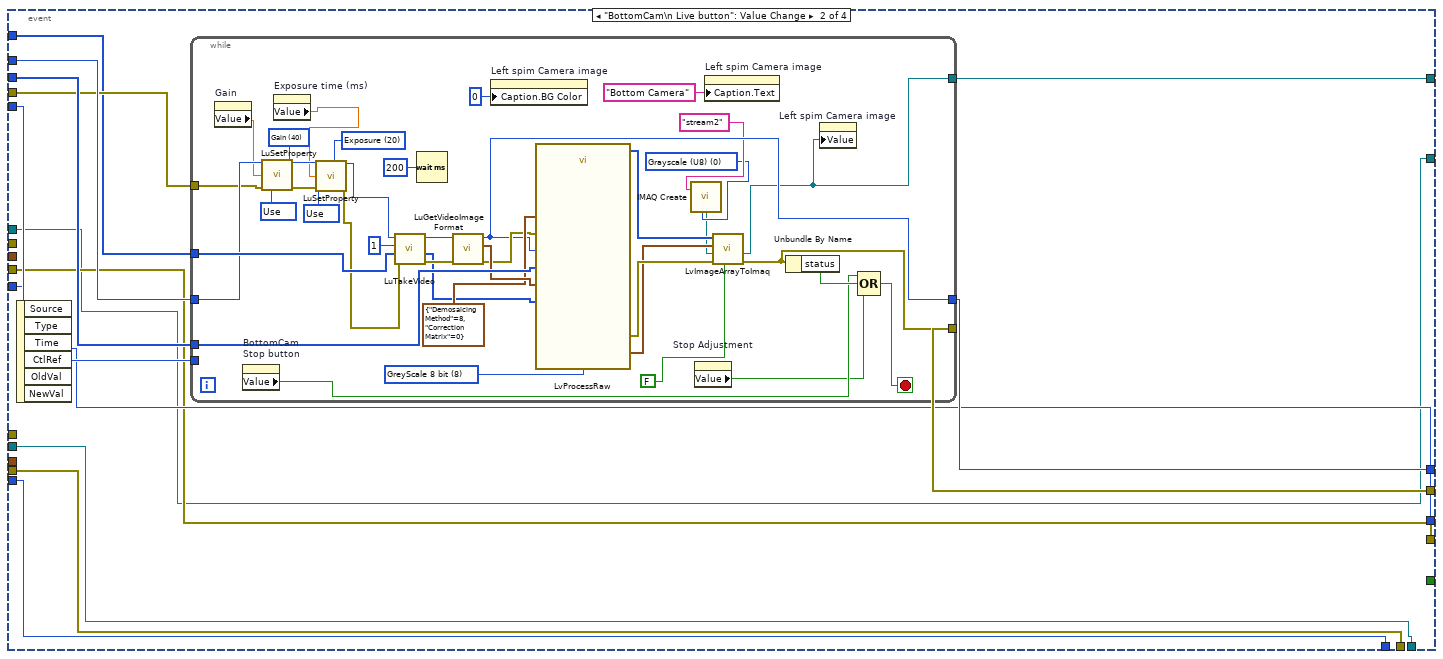
[diagram p17: hidden frame]
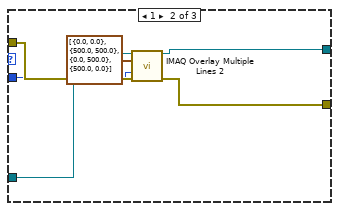
[diagram p19: hidden frame]
diagram:
  w63 = T9 {"Y-Gal ampl"=0.0, "A Z-Gal amp"=0.0, "A Z-Gal Off"=0.0, "Imag Obj Amp"=0.0, "A Obj Off H"=0.0, "A Obj Off L"=0.0, "B Obj Off H"=0.0, "B Obj Off L"=0.0, "B Z-Gal Amp"=0.0, "B Z-Gal Off"=0.0, "488 laser pow"=0.0, "561 laser pow"=0.0, "A Y-Gal Off"=0.0, "B Y-Gal Off "=0.0, "planes/vol"=0.0, "Time/plane"=0.0}  # Cluster_constant init
  # "File path for saving images in Hamamatsu format\nin Solid State Drive"
  # "SPIMB"
  # "SPIMA"
  n1 = Multiply(x="Z Step Size", y="Z-Galvo Conversion \nFactor B (V)") -> (x*y=w73:dbl)
  n2 = Multiply(x="Z Step Size", y="Piezo Conversion Factor (V)") -> (x*y=w30:dbl)
  n3 = Divide(x="# Planes/Volume", y=2.0) -> (x/y=w82:dbl)
  n4 = Multiply(x=w73, y=w82) -> (x*y=w83:dbl)
  n5 = Multiply(x=w82, y=w30) -> (x*y=w59:dbl)
  n6 = local read "AutoFocus \n(move only piezo)"() -> (w72:bool)
  n7 = Subtract(x="Z-Galvo Offset B (V)", y=w83) -> (x-y=w47:dbl)
  n8 = property on="Autofocus \n(move only galvo )" class="Bool (strict)"() -> ("Value"=w32:bool)  [unwired: 2 in, 2 out]
  n9 = Multiply(x="Z Step Size", y="Z-Galvo Conversion \nFactor A (V)") -> (x*y=w57:dbl)
  n10 = property on="AutoFocus \n(move only piezo)" class="Bool (strict)"() -> ("Value"=w43:bool)  [unwired: 2 in, 2 out]
  n11 = Add(x="Imaging Piezo Offset (V)\n(SPIM ARM A)", y=w59) -> (x+y=w41:dbl)
  n12 = Subtract(x="Imaging Piezo Offset (V)\n(SPIM ARM A)", y=w59) -> (x-y=w39:dbl)
  n13 = Add(x="Imaging Piezo Offset (V)\n(SPIM ARM B)", y=w59) -> (x+y=w37:dbl)
  n14 = Subtract(x="Imaging Piezo Offset (V)\n(SPIM ARM B)", y=w59) -> (x-y=w35:dbl)
  n15 = Multiply(x=w57, y=w82) -> (x*y=w84:dbl)
  n16 = case shown="False" w72 {
    tunnel: [w89 w90] -> w61
    tunnel: w73 -> [w89 _]
    tunnel: [w88 w90] -> w58
    tunnel: w57 -> [w88 _]
    frame False {
    }
    frame True {
      w90 = 0
    }
  }
  n17 = Subtract(x="Z-Galvo Offset A (V)", y=w84) -> (x-y=w46:dbl)
  n18 = case shown="False" w32 {
    tunnel: [w95 w98] -> w42
    tunnel: w41 -> [w95 _]
    tunnel: [w94 w98] -> w40
    tunnel: w39 -> [w94 _]
    tunnel: [w93 w97] -> w38
    tunnel: w37 -> [w93 _]
    tunnel: [w92 w97] -> w36
    tunnel: w35 -> [w92 _]
    tunnel: "Imaging Piezo Offset (V)\n(SPIM ARM A)" -> [_ w98]
    tunnel: "Imaging Piezo Offset (V)\n(SPIM ARM B)" -> [_ w97]
    tunnel: [w91 0.0] -> w31
    tunnel: w30 -> [w91 _]
    frame False {
    }
    frame True {
    }
  }
  n19 = case shown="False" w43 {
    tunnel: [w100 w102] -> w48
    tunnel: w47 -> [w100 _]
    tunnel: "Z-Galvo Offset B (V)" -> [_ w102]
    tunnel: w46 -> [w99 _]
    tunnel: [w99 w101] -> w45
    tunnel: "Z-Galvo Offset A (V)" -> [_ w101]
    frame False {
    }
    frame True {
    }
  }
  n20 = property on="Time/Plane" class="DigNum (strict)"() -> ("Value"=w20:dbl)  [unwired: 2 in, 2 out]
  n21 = property on="Z Step Size" class="DigNum (strict)"() -> ("Value"=w18:dbl)  [unwired: 2 in, 2 out]
  n22 = property on="# Planes/Volume" class="DigNum (strict)"() -> ("Value"=w16:dbl)  [unwired: 2 in, 2 out]
  n23 = property on="Light Sheet Width" class="DigNum (strict)"() -> ("Value"=w15:dbl)  [unwired: 2 in, 2 out]
  n24 = property on="Laser power (488 nm)" class="Slide (strict)"() -> ("Value"=w14:dbl)  [unwired: 2 in, 2 out]
  n25 = property on="Piezo Conversion Factor (V)" class="DigNum (strict)"() -> ("Value"=w4:dbl)  [unwired: 2 in, 2 out]
  n26 = property on="Laser power (561 nm)" class="Slide (strict)"() -> ("Value"=w13:dbl)  [unwired: 2 in, 2 out]
  n27 = property on="Z-Galvo Offset B (V)" class="DigNum (strict)"() -> ("Value"=w11:dbl)  [unwired: 2 in, 2 out]
  n28 = property on="Z-Galvo Conversion \nFactor A (V)" class="DigNum (strict)"() -> ("Value"=w10:dbl)  [unwired: 2 in, 2 out]
  n29 = property on="Imaging Piezo Offset (V)\n(SPIM ARM A)" class="DigNum (strict)"() -> ("Value"=w5:dbl)  [unwired: 2 in, 2 out]
  n30 = property on="Z-Galvo Offset A (V)" class="DigNum (strict)"() -> ("Value"=w12:dbl)  [unwired: 2 in, 2 out]
  n31 = property on="Z-Galvo Conversion \nFactor B (V)" class="DigNum (strict)"() -> ("Value"=w9:dbl)  [unwired: 2 in, 2 out]
  n32 = property on="Y-Galvo Offset A (V)" class="DigNum (strict)"() -> ("Value"=w8:dbl)  [unwired: 2 in, 2 out]
  n33 = property on="Imaging Piezo Offset (V)\n(SPIM ARM B)" class="DigNum (strict)"() -> ("Value"=w6:dbl)  [unwired: 2 in, 2 out]
  n34 = property on="Y-Galvo Offset B (V)" class="DigNum (strict)"() -> ("Value"=w7:dbl)  [unwired: 2 in, 2 out]
  n35 = Multiply(x="Light Sheet Width", y=0.012) -> (x*y=w62:dbl)
  n36 = Bundle By Name(cluster=T8 {"cTime/plane"=0.0, "cNoOfVol"=0.0, "cZStepSize"=0.0, "cTimePointDelay"=0.0, "cPlanes/Vol"=0.0, "cLightShtWdth"=0.0, "cLasPow488"=0.0, "cLasPow561"=0.0, "cZGalOffA"=0.0, "cZGalOffB"=0.0, "cZGalConvFacA"=0.0, "cZGalConvFacB"=0.0, "cYGalOffA"=0.0, "cYGalOffB"=0.0, "cPzOffB"=0.0, "cPzOffA"=0.0, "cPzConvFac"=0.0}, "cTime/plane"=w20, "cNoOfVol"="# of Volumes", "cZStepSize"=w18, "cTimePointDelay"="Time Point Delay", "cPlanes/Vol"=w16, "cLightShtWdth"=w15, "cLasPow488"=w14, "cLasPow561"=w13, "cZGalOffA"=w12, "cZGalOffB"=w11, "cZGalConvFacA"=w10, "cZGalConvFacB"=w9, "cYGalOffA"=w8, "cYGalOffB"=w7, "cPzOffB"=w6, "cPzOffA"=w5, "cPzConvFac"=w4) -> (w2:T8)
  n37 = Bundle By Name(cluster=w63, "Y-Gal ampl"=w62, "A Z-Gal amp"=w58, "A Z-Gal Off"=w45, "Imag Obj Amp"=w31, "A Obj Off H"=w42, "A Obj Off L"=w40, "B Obj Off H"=w38, "B Obj Off L"=w36, "B Z-Gal Amp"=w61, "B Z-Gal Off"=w48, "488 laser pow"="Laser power (488 nm)", "561 laser pow"="Laser power (561 nm)", "A Y-Gal Off"="Y-Galvo Offset A (V)", "B Y-Gal Off"="Y-Galvo Offset B (V)", "planes/vol"="# Planes/Volume", "Time/plane"="Time/Plane") -> (w60:T9)
  n38 = property on="File Path to save DCIMG files" class="Path"() -> ("Value"=w22:path)  [unwired: 2 in, 2 out]
  n39 = property on="Prefix for image filenames" class="Str"() -> ("Value"=w21:string)  [unwired: 2 in, 2 out]
  n40 = call "Initialize_TIGER_module.vi"() -> ("error out"=w67:errorcluster, "Status readout"=→"Scanner/Piezo \ncontrol mode":string)  [unwired: 10 in]
  n41 = Concatenate Strings(w21, "_bgnd" ("string")) -> (w27:string)
  n42 = call "Create_folders_for_SPIM_storage.vi"("Prefix for image filenames"=w27, "File Path to save DCIMG files"=w22) -> ("Arm1 path"=w24:path, "SpimA path"=w26:path, "SpimB path"=w25:path, "Arm2 path"=w23:path)  [unwired: 6 in]
  n43 = call "Create_folders_for_SPIM_storage.vi"("Prefix for image filenames"=w21, "File Path to save DCIMG files"=w22) -> ("Arm1 path"=w65:path, "SpimA path"=w64:path, "SpimB path"=w71:path, "Arm2 path"=w68:path)  [unwired: 6 in]
  "TIFF storage for SPIM ARM B" <- w68
  "TIFF storage for SPIM ARM A" <- w65
  n44 = case shown="\"Image Acquisition - Single Color\"" "Control Mode:" {
    tunnel: "Camera SPIMA" -> [_ w863 w1176]
    tunnel: "Camera SPIMB" -> [_ w862 w1175]
    tunnel: w64 -> [_ w860 w1173]
    tunnel: w71 -> [_ w861 w1174]
    tunnel: [_ w859 w1168] -> w81
    tunnel: [_ w858 w1167] -> w78
    tunnel: w71 -> [_ w849 w1154]
    tunnel: w64 -> [_ w850 w1155]
    tunnel: [w109 w844 w1149] -> w70
    tunnel: w65 -> [_ w842 w1147]
    tunnel: w68 -> [_ w841 w1146]
    tunnel: w67 -> [w156 w812 w1141]
    tunnel: w60 -> [w158 w826 w1145]
    tunnel: [w145 _ _] -> w50
    tunnel: [w157 _ _] -> w49
    tunnel: w26 -> [_ w828 _]
    tunnel: w25 -> [_ w827 _]
    tunnel: w26 -> [_ w816 _]
    tunnel: w25 -> [_ w815 _]
    tunnel: w24 -> [_ w814 _]
    tunnel: w23 -> [_ w813 _]
    tunnel: w22 -> [_ w811 w1133]
    tunnel: w21 -> [_ w810 w1132]
    tunnel: w2 -> [_ w805 w1135]
    tunnel: [_ w803 w1134] -> w1
    frame "Parameter Adjustment" {
      w180 = 10158 items=["Allow Regeneration"=10097, "Do Not Allow Regeneration"=10158] ("RegenMode")
      w196 = 10158 items=["Allow Regeneration"=10097, "Do Not Allow Regeneration"=10158] ("RegenMode")
      n45 = property on="Camera SPIMA" class="Clust (strict)"() -> ("Value"=w125:T7)  [unwired: 2 in, 2 out]
      n46 = property on="Laser beam reference" class="Ring (strict)" props=["Value"]() -> ()  [unwired: 2 in, 3 out]
      n47 = property on="Camera SPIMB" class="Clust (strict)"() -> ("Value"=w126:T7)  [unwired: 2 in, 2 out]
      n48 = property on="Exposure time (ms)" class="Slide (strict)"() -> ("Value"=w155:sgl)  [unwired: 2 in, 2 out]
      n49 = property on="Gain" class="Slide (strict)"() -> ("Value"=w154:sgl)  [unwired: 2 in, 2 out]
      n50 = call "initialize_SPIMCams_Param_Adjust_(SubVI).vi"("Image Name"="stream 2", "Cam A ROI"=w126, "Cam B ROI"=w125, "Camera select"=u16 0) -> ("error out"=w121:errorcluster, "Buffer Info"=w120:T12, "IMAQ error out"=w118:errorcluster, "IMAQ image out"=w119:T6, "Handle out"=w122:u32, "Camera Details"=→"Camera 2 Details":T5)  [unwired: 2 in]
      n51 = call "initialize_SPIMCams_Param_Adjust_(SubVI).vi"("Image Name"="stream 1", "Cam A ROI"=w126, "Cam B ROI"=w125, "Camera select"=u16 1) -> ("error out"=w140:errorcluster, "Buffer Info"=w141:T12, "IMAQ error out"=w142:errorcluster, "IMAQ image out"=w143:T6, "Handle out"=w139:u32, "Camera Details"=→"Camera 1 Details":T5)  [unwired: 2 in]
      n52 = call "intialize_bottom_cam (SubVI).vi"("Gain"=w154, "Exposure time (ms)"=w155) -> ("images array out"=w150:u8[], "Handle out"=w153:u64, "BGR out"=w152:u8[], "Pixel Format"=w149:u32, "error out"=w151:errorcluster)  [unwired: 9 in]
      n53 = while {
        tunnel: [w419] -> w131
        tunnel: w153 -> [w415]
        tunnel: w152 -> [w414]
        tunnel: w151 -> [w413]
        tunnel: w150 -> [w412]
        tunnel: w149 -> [w411]
        tunnel: [w410] -> w146
        tunnel: w143 -> [w409]
        tunnel: w142 -> [w408]
        tunnel: w141 -> [w407]
        tunnel: w140 -> [w406]
        tunnel: w139 -> [w405]
        tunnel: [w404] -> w128
        tunnel: [w403] -> w133
        tunnel: [w402] -> w132
        tunnel: [w401] -> w129
        tunnel: w122 -> [w400]
        tunnel: w121 -> [w399]
        tunnel: w120 -> [w398]
        tunnel: w119 -> [w397]
        tunnel: w118 -> [w396]
        tunnel: [w395] -> w112
        tunnel: [w394] -> w108
        tunnel: [w393] -> w106
        stop <- w416 stop-if-true
        n54 = event shown="[2] \"Start SPIM  live\": Value Change" {
          selector: _ -> [_ _ _ _]
          dyn-events: _ -> [_ _ _ _]
          timeout: -1 -> [_ _ _ _]
          tunnel: [w426 w435 w490 w675] -> w419
          tunnel: [_ _ _ TRUE] -> w416
          tunnel: w415 -> [w427 w441 w491 w674]
          tunnel: w414 -> [_ w440 _ _]
          tunnel: w413 -> [w426 w439 w490 w675]
          tunnel: w412 -> [_ w438 _ _]
          tunnel: w411 -> [_ w437 _ _]
          tunnel: [w427 w436 w491 w674] -> w410
          tunnel: w409 -> [w421 w429 w498 w671]
          tunnel: w408 -> [_ _ w497 _]
          tunnel: w407 -> [_ _ w496 _]
          tunnel: w406 -> [w425 w433 w495 w676]
          tunnel: w405 -> [w424 w434 w494 w677]
          tunnel: [w425 w433 w493 w676] -> w404
          tunnel: [w424 w434 w492 w677] -> w403
          tunnel: [_ w432 _ _] -> w402
          tunnel: [w421 w429 w489 w671] -> w401
          tunnel: w400 -> [w423 w431 w488 w673]
          tunnel: w399 -> [w422 w430 w487 w672]
          tunnel: w398 -> [_ _ w486 _]
          tunnel: w397 -> [w420 w428 w485 w670]
          tunnel: w396 -> [_ _ w484 _]
          tunnel: [w423 w431 w483 w673] -> w395
          tunnel: [w422 w430 w482 w672] -> w394
          tunnel: [w420 w428 w481 w670] -> w393
          event Timeout {
            n55 = event-data() -> ()  [unwired: 1 in, 3 out]
          }
          event "BottomCam\n Live button": Value Change {
            n56 = event-data() -> ()  [unwired: 1 in, 6 out]
            n57 = while {
              tunnel: w438 -> [w480]
              tunnel: w440 -> [w479]
              tunnel: w437 -> [_]
              tunnel: w441 -> [w464]
              tunnel: [w467] -> w436
              tunnel: w439 -> [w461]
              tunnel: [w466] -> w435
              tunnel: [w447] -> w432
              stop <- w465 stop-if-true
              w448 = u32 8 items=["8 Bit raw", "16 Bit raw", "RGB 24", "YUV422", "COUNT", "FILTER", "RGB 32", "RGB 48", "GreyScale 8 bit", "GreyScale 16 bit"] ("Pixel Format")
              w449 = T13 0 items=["Grayscale (U8)", "Grayscale (I16)", "Grayscale (SGL)", "Complex (CSG)", "RGB (U32)", "HSL (U32)", "RGB (U64)", "Grayscale (U16)"] ("Image Type")
              w455 = T14 20 items=["Contrast"=1, "Hue"=2, "Brightness"=0, "Saturation"=3, "Sharpness"=4, "Gamma"=5, "Pan"=16, "Tilt"=17, "Roll"=18, "Zoom"=19, "Exposure"=20, "Iris"=21, "Focus"=22, "Gain"=40, "Gain Red/Magenta"=41, "Gain Blue/Cyan"=42, "Gain Green1/Yellow1"=43, "Gain Green2/Yellow2"=44, "Still Exposure"=50, "Still Gain"=51, "Red Still Gain"=52, "Green1 Still Gain"=53, "Green2 Still Gain"=54, "Blue Still Gain"=55, "Still Strobe Delay"=56, "Still Exposure Delay"=100, "Demosaicing Method"=64, "Correction Matrix"=65, "Flipping"=66, "Digital Whitebalance U"=69, "Digital Whitebalance V"=70, "Digital Gain"=71, "Digital Gain Red"=72, "Digital Gain Green"=73, "Digital Gain Blue"=74, "Color Format"=80, "Max Width"=81, "Max Height"=82, "ABS Focus"=85, "Black Level"=86, "Still Knee1 Exposure"=96, "Still Knee2 Exposure"=97, "Still Knee3 Exposure"=98, "Video Knee"=99, "Threshold"=101, "Auto Exp Target"=103, "Timestamps"=105, "Snapshot Clock Speed"=106, "Auto Exp Maximum"=107, "Temperature"=108, "Trigger"=110, "Frame Gate"=112, "Exposure Interval"=113, "PWM"=114, "Memory"=115, "Still Strobe Duration"=116, "Fan"=118, "Sync Mode"=119, "Snapshot Count"=120, "LSC X"=121, "LSC Y"=122, "Auto Iris Max"=123, "Lens Stabilization"=124, "Video Trigger"=125, "Knee2 Level"=163, "Threshold Low"=165, "Threshold High"=166, "Temperature2"=167, "Light Frequency"=168, "Luminance"=169, "Auto Gain Max"=170, "Focal Length"=174, "Iris Latency"=175, "TAP Video Configuration"=176, "TAP Still Configuration"=177, "JPEG Quality"=256, "GEV LLA"=512, "GEV DHCP"=513, "GEV PERSISTANT"=514, "GEV PERSISTANT IP Addrress"=515, "GEV PERSISTANT IP Subnet Mask"=516, "GEV PERSISTANT Default Gateway"=517, "GEV  SCPD"=518] ("Property")
              w456 = T14 40 items=["Contrast"=1, "Hue"=2, "Brightness"=0, "Saturation"=3, "Sharpness"=4, "Gamma"=5, "Pan"=16, "Tilt"=17, "Roll"=18, "Zoom"=19, "Exposure"=20, "Iris"=21, "Focus"=22, "Gain"=40, "Gain Red/Magenta"=41, "Gain Blue/Cyan"=42, "Gain Green1/Yellow1"=43, "Gain Green2/Yellow2"=44, "Still Exposure"=50, "Still Gain"=51, "Red Still Gain"=52, "Green1 Still Gain"=53, "Green2 Still Gain"=54, "Blue Still Gain"=55, "Still Strobe Delay"=56, "Still Exposure Delay"=100, "Demosaicing Method"=64, "Correction Matrix"=65, "Flipping"=66, "Digital Whitebalance U"=69, "Digital Whitebalance V"=70, "Digital Gain"=71, "Digital Gain Red"=72, "Digital Gain Green"=73, "Digital Gain Blue"=74, "Color Format"=80, "Max Width"=81, "Max Height"=82, "ABS Focus"=85, "Black Level"=86, "Still Knee1 Exposure"=96, "Still Knee2 Exposure"=97, "Still Knee3 Exposure"=98, "Video Knee"=99, "Threshold"=101, "Auto Exp Target"=103, "Timestamps"=105, "Snapshot Clock Speed"=106, "Auto Exp Maximum"=107, "Temperature"=108, "Trigger"=110, "Frame Gate"=112, "Exposure Interval"=113, "PWM"=114, "Memory"=115, "Still Strobe Duration"=116, "Fan"=118, "Sync Mode"=119, "Snapshot Count"=120, "LSC X"=121, "LSC Y"=122, "Auto Iris Max"=123, "Lens Stabilization"=124, "Video Trigger"=125, "Knee2 Level"=163, "Threshold Low"=165, "Threshold High"=166, "Temperature2"=167, "Light Frequency"=168, "Luminance"=169, "Auto Gain Max"=170, "Focal Length"=174, "Iris Latency"=175, "TAP Video Configuration"=176, "TAP Still Configuration"=177, "JPEG Quality"=256, "GEV LLA"=512, "GEV DHCP"=513, "GEV PERSISTANT"=514, "GEV PERSISTANT IP Addrress"=515, "GEV PERSISTANT IP Subnet Mask"=516, "GEV PERSISTANT Default Gateway"=517, "GEV  SCPD"=518] ("Property")
              w457 = -2147483648 items=["None"=0, "Use"=-2147483648, "Auto\\Master\\Little Endian"=1073741824, "Strobe From Start of Exposure"=536870912, "Polarity"=268435456, "Memory Readback"=134217728, "Unknown Maximum"=131072, "Unknown Minimum"=65536, "Red"=1, "Green1"=2, "Green2"=4, "Blue"=8] ("Capability Flag")
              w458 = -2147483648 items=["None"=0, "Use"=-2147483648, "Auto\\Master\\Little Endian"=1073741824, "Strobe From Start of Exposure"=536870912, "Polarity"=268435456, "Memory Readback"=134217728, "Unknown Maximum"=131072, "Unknown Minimum"=65536, "Red"=1, "Green1"=2, "Green2"=4, "Blue"=8] ("Capability Flag")
              n58 = property on="Gain" class="Slide (strict)"() -> ("Value"=w454:sgl)  [unwired: 2 in, 2 out]
              n59 = property on="BottomCam \nStop button" class="Bool (strict)"() -> ("Value"=w453:bool)  [unwired: 2 in, 2 out]
              n60 = call <userlib>:"LuSetProperty.vi"("handle in"=w464, "Property"=w456, "value"=w454, "Capability Flag"=w458, "error in (no error)"=w461) -> ("Handle out"=w463:u64, "error out"=w460:errorcluster)  [unwired: 9 in]
              n61 = property on="Exposure time (ms)" class="Slide (strict)"() -> ("Value"=w443:sgl)  [unwired: 2 in, 2 out]
              n62 = call <userlib>:"LuSetProperty.vi"("handle in"=w463, "Property"=w455, "value"=w443, "Capability Flag"=w457, "error in (no error)"=w460) -> ("Handle out"=w462:u64, "error out"=w459:errorcluster)  [unwired: 9 in]
              n63 = call <userlib>:"LuTakeVideo.vi"("error in"=w459, "Image In"=w480, "frame count"=1, "handle in"=w462) -> ("error out"=w477:errorcluster, "Image out"=w451:u8[], "handle out"=w476:u64)  [unwired: 3 in]
              n64 = Wait (ms)(milliseconds to wait=u32 200) -> ()  [unwired: 1 out]
              n65 = call <userlib>:"LuGetVideoImageFormat.vi"("error in"=w477, "handle in"=w476) -> ("error out"=w473:errorcluster, "image format"=w475:T15, "handle out"=w467:u64)  [unwired: 7 in]
              n66 = property on="Left spim Camera image" class="ImageControl"("Caption.BG Color"=u32 0 ("Caption.Colors:BG Color")) -> ()  [unwired: 2 in, 2 out]
              n67 = call <userlib>:"LvProcessRaw.vi"("handle in"=w467, "ImageRaw"=w451, "Image Format"=w475, "Image BGR in"=w479, "Pixel Format"=w448, "CONVERSION"=T10 {"Demosaicing Method"=8, "Correction Matrix"=0}, "error in"=w473) -> ("image out"=w470:u8[], "Image Format out"=w471:T15, "error out"=w472:errorcluster)  [unwired: 17 in, 1 out]
              n68 = call "IMAQ Create"("Image Name"="stream2", "Image Type"=w449) -> ("New Image"=w446:T6)  [unwired: 3 in, 1 out]
              n69 = property on="Stop Adjustment" class="Bool (strict)"() -> ("Value"=w452:bool)  [unwired: 2 in, 2 out]
              n70 = property on="Left spim Camera image" class="ImageControl"("Caption.Text"="Bottom Camera") -> ()  [unwired: 2 in, 2 out]
              n71 = call <userlib>:"LvImageArrayToImaq.vi"("IsBigEndian"=FALSE, "error in"=w472, "Imaq Image"=w446, "Image Format"=w471, "image converted"=w470) -> ("error out"=w466:errorcluster, "Image Out"=w447:T16)  [unwired: 5 in]
              n72 = Unbundle By Name(w466) -> ("status"=w468:bool)
              n73 = property on="Left spim Camera image" class="ImageControl"("Value"=w447) -> ()  [unwired: 2 in, 2 out]
              n74 = Compound Arithmetic op=OR(w453, w468, w452) -> (w465:bool)
            }
          }
          event "Start SPIM \nlive": Value Change {
            n75 = event-data() -> ()  [unwired: 1 in, 6 out]
            n76 = while {
              tunnel: w495 -> [w576]
              tunnel: w496 -> [w518]
              tunnel: [w554] -> w493
              tunnel: w498 -> [w511]
              tunnel: w497 -> [w514]
              tunnel: w494 -> [w577]
              tunnel: [w572] -> w492
              tunnel: [w501] -> w489
              tunnel: w488 -> [w553]
              tunnel: w487 -> [w552]
              tunnel: w486 -> [w528]
              tunnel: w485 -> [w523]
              tunnel: w484 -> [w526]
              tunnel: [w535] -> w483
              tunnel: [w534] -> w482
              tunnel: [w508] -> w481
              stop <- w570 stop-if-true
              n77 = flat-sequence {
                tunnel: w577 -> [w611]
                tunnel: w576 -> [w610]
                tunnel: [w609] -> w575
                tunnel: [w608] -> w574
                tunnel: [w597] -> w573
                tunnel: w553 -> [w607]
                tunnel: w552 -> [w606]
                tunnel: [w605] -> w551
                tunnel: [w604] -> w550
                tunnel: [w596] -> w529
                tunnel: w528 -> [w603]
                tunnel: [w603] -> w527
                tunnel: w526 -> [w602]
                tunnel: [w602] -> w525
                tunnel: w523 -> [w601]
                tunnel: [w601] -> w522
                tunnel: [w600] -> w519
                tunnel: w518 -> [w600]
                tunnel: [w599] -> w515
                tunnel: w514 -> [w599]
                tunnel: [w598] -> w512
                tunnel: w511 -> [w598]
                frame #0 {
                  n78 = call <userlib>:"tm_waitnextframe_40.vi"("error in (no error)"=w606, "Handle in"=w607) -> ("error out"=w605:errorcluster, "Frame Index"=w596:i32, "Handle out"=w604:u32)  [unwired: 6 in, 1 out]
                  n79 = call <userlib>:"tm_waitnextframe_40.vi"("error in (no error)"=w610, "Handle in"=w611) -> ("error out"=w608:errorcluster, "Frame Index"=w597:i32, "Handle out"=w609:u32)  [unwired: 6 in, 1 out]
                }
              }
              n80 = property on="Overlay Color" class="ColBox"() -> ("Value"=w536:u32)  [unwired: 2 in, 2 out]
              n81 = flat-sequence {
                tunnel: w575 -> [w583]
                tunnel: w574 -> [w582]
                tunnel: w573 -> [w581]
                tunnel: [w579] -> w572
                tunnel: [w578] -> w569
                tunnel: w519 -> [w586]
                tunnel: [w580] -> w554
                tunnel: w551 -> [w595]
                tunnel: w550 -> [w594]
                tunnel: [w593] -> w549
                tunnel: w527 -> [w587]
                tunnel: [w592] -> w535
                tunnel: [w591] -> w534
                tunnel: w529 -> [w590]
                tunnel: w525 -> [w589]
                tunnel: [w589] -> w524
                tunnel: w522 -> [w588]
                tunnel: [w588] -> w521
                tunnel: [w587] -> w520
                tunnel: [w586] -> w517
                tunnel: [w585] -> w516
                tunnel: w515 -> [w585]
                tunnel: [w584] -> w513
                tunnel: w512 -> [w584]
                frame #0 {
                  n82 = call <userlib>:"tm_getframe16_40.vi"("error in (no error)"=w582, "Frame Index"=w581, "Handle in"=w583) -> ("error out"=w580:errorcluster, "Data"=w578:u16[][], "Handle out"=w579:u32)  [unwired: 5 in, 1 out]
                  n83 = call <userlib>:"tm_getframe16_40.vi"("error in (no error)"=w595, "Frame Index"=w590, "Handle in"=w594) -> ("error out"=w591:errorcluster, "Data"=w593:u16[][], "Handle out"=w592:u32)  [unwired: 5 in, 1 out]
                }
              }
              n84 = property on="higher threshold" class="Slide (strict)"() -> ("Value"=w509:u16)  [unwired: 2 in, 2 out]
              n85 = property on="mid-level" class="Slide (strict)"() -> ("Value"=w499:u16)  [unwired: 2 in, 2 out]
              n86 = property on="lower threshold" class="Slide (strict)"() -> ("Value"=w510:u16)  [unwired: 2 in, 2 out]
              n87 = call "IMAQ ArrayToImage"("Image Pixels (U16)"=w549, "error in (no error)"=w524, "Image"=w521) -> ("error out"=w540:errorcluster, "Image Out"=w538:T6)  [unwired: 7 in]
              n88 = call "IMAQ ArrayToImage"("Image Pixels (U16)"=w569, "error in (no error)"=w516, "Image"=w513) -> ("error out"=w567:errorcluster, "Image Out"=w568:T6)  [unwired: 7 in]
              n89 = Unbundle By Name(w520) -> ("height"=w542:u32, "width"=w541:u32)
              n90 = Divide(x=w542, y=u32 2) -> (x/y=w544:dbl)
              n91 = Unbundle By Name(w517) -> ("height"=w556:u32, "width"=w555:u32)
              n92 = Build Array(0.0 ("element"), w544, w541, w544) -> (w545:dbl[])
              n93 = Divide(x=w556, y=u32 2) -> (x/y=w558:dbl)
              n94 = call "IMAQ LineProfile"("error in (no error)"=w540, "Line Coordinates"=w545, "Image"=w538) -> ("error out"=w537:errorcluster, "Line Graph"=w548:cluster{"x0":sgl, "dx":sgl, "Pixels Line":sgl[]})  [unwired: 2 in, 2 out]
              n95 = call "adjustable_lookup_for_image_display (SubVI).vi"("Mid-level value"=w499, "Minimum value"=w510, "Maximum value"=w509) -> ("User-defined Look-up table"=w502:u16[])  [unwired: 8 in]
              n96 = Build Array(0.0 ("element"), w558, w555, w558) -> (w559:dbl[])
              n97 = Unbundle By Name(w548) -> ("Pixels Line"=→"Waveform Graph 2":sgl[])  [unwired: 2 out]
              n98 = call "IMAQ LineProfile"("error in (no error)"=w567, "Line Coordinates"=w559, "Image"=w568) -> ("error out"=w566:errorcluster, "Line Graph"=w565:cluster{"x0":sgl, "dx":sgl, "Pixels Line":sgl[]})  [unwired: 2 in, 2 out]
              n99 = Unbundle By Name(w565) -> ("Pixels Line"=→"Waveform Graph":sgl[])  [unwired: 2 out]
              n100 = case shown="2" "Choose Overlay" {
                tunnel: w538 -> [w613 w619 w640]
                tunnel: [w613 w618 w635] -> w508
                tunnel: w537 -> [w612 w617 w639]
                tunnel: [w612 w616 w637] -> w506
                tunnel: w536 -> [_ w614 w634]
                tunnel: w542 -> [_ _ w623]
                tunnel: w541 -> [_ _ w620]
                frame 0, Default {
                }
                frame 1 {
                  n101 = call "IMAQ Overlay Multiple Lines 2"("Image"=w619, "Line End Points"=cluster{"X":dbl, "Y":dbl}[] [{"X"=0.0, "Y"=0.0}, {"X"=500.0, "Y"=500.0}, {"X"=0.0, "Y"=500.0}, {"X"=500.0, "Y"=0.0}], "Color"=w614, "error in (no error)"=w617) -> ("Image Out"=w618:T6, "error out"=w616:errorcluster)  [unwired: 10 in]
                }
                frame 2 {
                  w633 = 0.0 ("element")
                  w630 = cluster{"element":dbl, dbl} {"element"=0.0, 0.0} ("cluster")
                  n102 = Divide(x=w623, y=2.0) -> (x/y=w621:dbl)
                  n103 = Divide(x=w620, y=u32 2) -> (x/y=w622:dbl)
                  n104 = Bundle(cluster=w630, "element"=w633, w621) -> (w628:cluster{"element":dbl, dbl})
                  n105 = Bundle(cluster=w630, "element"=w620, w621) -> (w629:cluster{"element":dbl, dbl})
                  n106 = Bundle(cluster=w630, "element"=w622, w633) -> (w631:cluster{"element":dbl, dbl})
                  n107 = Bundle(cluster=w630, "element"=w622, w620) -> (w632:cluster{"element":dbl, dbl})
                  n108 = Build Array(w628, w629) -> (w627:cluster{"element":dbl, dbl}[])
                  n109 = call "IMAQ Overlay Multiple Lines 2"("Image"=w640, "Line End Points"=w627, "Color"=w634, "error in (no error)"=w639) -> ("Image Out"=w636:T6, "error out"=w638:errorcluster)  [unwired: 10 in]
                  n110 = Build Array(w631, w632) -> (w626:cluster{"element":dbl, dbl}[])
                  n111 = call "IMAQ Overlay Multiple Lines 2"("Image"=w636, "Line End Points"=w626, "Color"=w634, "error in (no error)"=w638) -> ("Image Out"=w635:T6, "error out"=w637:errorcluster)  [unwired: 10 in]
                }
              }
              n112 = case shown="2" "Choose Overlay" {
                tunnel: w568 -> [w642 w648 w669]
                tunnel: [w642 w647 w664] -> w501
                tunnel: w566 -> [w641 w646 w668]
                tunnel: [w641 w645 w666] -> w504
                tunnel: w536 -> [_ w643 w663]
                tunnel: w556 -> [_ _ w652]
                tunnel: w555 -> [_ _ w649]
                frame 0, Default {
                }
                frame 1 {
                  n113 = call "IMAQ Overlay Multiple Lines 2"("Image"=w648, "Line End Points"=cluster{"X":dbl, "Y":dbl}[] [{"X"=0.0, "Y"=0.0}, {"X"=500.0, "Y"=500.0}, {"X"=0.0, "Y"=500.0}, {"X"=500.0, "Y"=0.0}], "Color"=w643, "error in (no error)"=w646) -> ("Image Out"=w647:T6, "error out"=w645:errorcluster)  [unwired: 10 in]
                }
                frame 2 {
                  w662 = 0.0 ("element")
                  w659 = cluster{"element":dbl, dbl} {"element"=0.0, 0.0} ("cluster")
                  n114 = Divide(x=w652, y=2.0) -> (x/y=w650:dbl)
                  n115 = Divide(x=w649, y=u32 2) -> (x/y=w651:dbl)
                  n116 = Bundle(cluster=w659, "element"=w662, w650) -> (w657:cluster{"element":dbl, dbl})
                  n117 = Bundle(cluster=w659, "element"=w649, w650) -> (w658:cluster{"element":dbl, dbl})
                  n118 = Bundle(cluster=w659, "element"=w651, w662) -> (w660:cluster{"element":dbl, dbl})
                  n119 = Bundle(cluster=w659, "element"=w651, w649) -> (w661:cluster{"element":dbl, dbl})
                  n120 = Build Array(w657, w658) -> (w656:cluster{"element":dbl, dbl}[])
                  n121 = call "IMAQ Overlay Multiple Lines 2"("Image"=w669, "Line End Points"=w656, "Color"=w663, "error in (no error)"=w668) -> ("Image Out"=w665:T6, "error out"=w667:errorcluster)  [unwired: 10 in]
                  n122 = Build Array(w660, w661) -> (w655:cluster{"element":dbl, dbl}[])
                  n123 = call "IMAQ Overlay Multiple Lines 2"("Image"=w665, "Line End Points"=w655, "Color"=w663, "error in (no error)"=w667) -> ("Image Out"=w664:T6, "error out"=w666:errorcluster)  [unwired: 10 in]
                }
              }
              n124 = call "IMAQ UserLookup 2"("Image Src"=w501, "Lookup Table"=w502, "error in (no error)"=w504) -> ("Image Dst Out"=w500:T6, "error out"=w503:errorcluster)  [unwired: 4 in]
              n125 = property on="Left spim Camera image" class="ImageControl"("Value"=w500) -> ()  [unwired: 2 in, 2 out]
              n126 = call "IMAQ UserLookup 2"("Image Src"=w508, "Lookup Table"=w502, "error in (no error)"=w506) -> ("Image Dst Out"=w507:T6, "error out"=w505:errorcluster)  [unwired: 4 in]
              n127 = property on="Right spim Camera image" class="ImageControl"("Caption.BGColor"=u32 0 ("Caption.Text Colors:BG Color")) -> ()  [unwired: 2 in, 2 out]
              n128 = property on="Right spim Camera image" class="ImageControl"("Value"=w507) -> ()  [unwired: 2 in, 2 out]
              n129 = property on="Right spim Camera image" class="ImageControl"("Caption.Text"="Right SPIM Cam") -> ()  [unwired: 2 in, 2 out]
              n130 = property on="Left spim Camera image" class="ImageControl"("Caption.Text"="Left SPIM Cam") -> ()  [unwired: 2 in, 2 out]
              n131 = property on="Left spim Camera image" class="ImageControl"("Caption.BG Color"=u32 0 ("Caption.Colors:BG Color")) -> ()  [unwired: 2 in, 2 out]
              n132 = Merge Errors(w503, w505) -> (w532:errorcluster)
              n133 = property on="Stop SPIM \nlive" class="Bool (strict)"() -> ("Value"=w563:bool)  [unwired: 2 in, 2 out]
              n134 = Unbundle By Name(w554) -> ("status"=w571:bool)
              n135 = Unbundle By Name(w534) -> ("status"=w533:bool)
              n136 = call <vilib>:"General Error Handler.vi"("error in (no error)"=w532) -> ()  [unwired: 10 in, 5 out]
              n137 = Compound Arithmetic op=OR(w571, w563, w533) -> (w570:bool)
            }
          }
          event "Stop Adjustment": Value Change {
            n138 = event-data() -> ()  [unwired: 1 in, 6 out]
          }
        }
        n139 = Wait (ms)(milliseconds to wait=u32 100) -> ()  [unwired: 1 out]
      }
      n140 = call-poly <vilib>:"DAQmx Create Virtual Channel.vi"("physical channels"=tag "PXI1Slot4/ao0:5") -> ("task out"=w193:refnum<k21>, "error out"=w192:errorcluster)  [unwired: 13 in]
      n141 = call-poly <vilib>:"DAQmx Create Virtual Channel.vi"("physical channels"=tag "PXI1Slot5/ao2:4") -> ("task out"=w182:refnum<k21>, "error out"=w181:errorcluster)  [unwired: 13 in]
      n142 = property class="DAQmx Write"(reference=w182, error in=w181, "Regeneration Mode"=w180) -> (reference out=w178:refnum<k21>, error out=w177:errorcluster)
      n143 = property class="DAQmx Write"(reference=w193, error in=w192, "Regeneration Mode"=w196) -> (reference out=w195:refnum<k21>, error out=w194:errorcluster)
      n144 = Bundle(cluster=cluster{"Fs":dbl, "#s":dbl} {"Fs"=1000.0, "#s"=1000.0} ("sampling info"), "Fs"=10000.0, "#s"=1000.0) -> (w159:cluster{"Fs":dbl, "#s":dbl})
      n145 = Bundle(cluster=cluster{"Fs":dbl, "#s":dbl} {"Fs"=1000.0, "#s"=1000.0} ("sampling info"), "Fs"=10000.0, "#s"=1000.0) -> (w189:cluster{"Fs":dbl, "#s":dbl})
      n146 = while {
        tunnel: w189 -> [w777]
        tunnel: w159 -> [w776]
        tunnel: [w773] -> w176
        tunnel: [w772] -> w175
        shift-right: [w779] -> w191
        shift-left: w195 -> [w781]
        shift-right: [w778] -> w190
        shift-left: w194 -> [w780]
        shift-right: [w771] -> w165
        shift-left: w178 -> [w775]
        shift-right: [w770] -> w164
        shift-left: w177 -> [w774]
        tunnel: w158 -> [w704]
        stop <- w703 stop-if-true
        w726 = 10123 items=["Finite Samples"=10178, "Continuous Samples"=10123, "Hardware Timed Single Point"=12522] ("sample mode")
        w761 = 10123 items=["Finite Samples"=10178, "Continuous Samples"=10123, "Hardware Timed Single Point"=12522] ("sample mode")
        # "1: ARM1  Z-Axis control Waveform\n2: ARM1 Y-Axis control Waveform\n3: Collection Objective Piezo (ARM2)\n4: ARM2 Z-axis\n5: ARM2 Y-Axis\n6: Excitation Objective Piezo (ARM1)\n1*: 488-nm Laser intensity\n2*: 561-nm Laser intensity\n3*: Laser blanking"
        # "3*"
        # "2*"
        # "1*"
        # "4"
        # "6"
        # "5"
        # "3"
        # "2"
        # "1"
        n147 = property on="SPIM camera \nselection" class="Ring (strict)"() -> ("Value"=w700:u16)  [unwired: 2 in, 2 out]
        n148 = property on="Z-galvo Offset A slider" class="Slide (strict)"() -> ("Value"=w686:dbl)  [unwired: 2 in, 2 out]
        n149 = case shown="0, Default" w700 {
          tunnel: [w785 w789] -> w697
          tunnel: [w784 w788] -> w696
          tunnel: [w783 w787] -> w690
          tunnel: [w782 w786] -> w689
          frame 0, Default {
            n150 = property on="Imaging \nscanning" class="Bool (strict)"() -> ("Value"=w783:bool)  [unwired: 2 in, 2 out]
            n151 = property on="Epi" class="Bool (strict)"() -> ("Value"=w784:bool)  [unwired: 2 in, 2 out]
            n152 = property on="Epi scanning" class="Bool (strict)"() -> ("Value"=w782:bool)  [unwired: 2 in, 2 out]
            n153 = property on="Imaging" class="Bool (strict)"() -> ("Value"=w785:bool)  [unwired: 2 in, 2 out]
          }
          frame 1 {
            n154 = property on="Epi" class="Bool (strict)"() -> ("Value"=w789:bool)  [unwired: 2 in, 2 out]
            n155 = property on="Imaging" class="Bool (strict)"() -> ("Value"=w788:bool)  [unwired: 2 in, 2 out]
            n156 = property on="Imaging \nscanning" class="Bool (strict)"() -> ("Value"=w786:bool)  [unwired: 2 in, 2 out]
            n157 = property on="Epi scanning" class="Bool (strict)"() -> ("Value"=w787:bool)  [unwired: 2 in, 2 out]
          }
        }
        n158 = Unbundle By Name(w704) -> ("Y-Gal ampl"=w692:dbl)
        n159 = property on="Z-Galvo Offset A (V)" class="DigNum (strict)"() -> ("Value"=w684:dbl)  [unwired: 2 in, 2 out]
        n160 = Multiply(x=w686, y=0.001) -> (x*y=w687:dbl)
        n161 = Add(x=w687, y=w684) -> (x+y=w685:dbl)
        n162 = Select(t=w692, s=w690, f=0.0) -> (s? t:f=w695:dbl)
        n163 = property on="Y-Galvo Offset A (V)" class="DigNum (strict)"() -> ("Value"=w705:dbl)  [unwired: 2 in, 2 out]
        n164 = Select(t=w685, s=w697, f=0.0) -> (s? t:f=w701:dbl)
        n165 = call <vilib>:"Basic Function Generator.vi"("offset"=w701, "square wave duty cycle (%)"=100.0, "sampling info"=w777, "signal type"=T11."Square Wave", "phase"=0.0, "amplitude"=0.0, "frequency"=10.0) -> ("signal out"=w727:waveform(dbl))  [unwired: 2 in, 2 out]
        n166 = call <vilib>:"Basic Function Generator.vi"("offset"=w705, "sampling info"=w776, "signal type"=T11."Triangle Wave", "phase"=0.0, "amplitude"=w695, "frequency"=100.0) -> ("signal out"=w764:waveform(dbl))  [unwired: 3 in, 2 out]
        n167 = call-poly <vilib>:"DAQmx Timing.vi"("task/channels in"=w781, "sample mode"=w761, "waveform"=w727, "error in"=w780) -> ("task out"=w763:refnum<k21>, "error out"=w762:errorcluster)  [unwired: 10 in]
        n168 = local read "Imaging Piezo Offset (V)\n(SPIM ARM B)"() -> (w709:dbl)
        n169 = call <vilib>:"Basic Function Generator.vi"("offset"=w709, "square wave duty cycle (%)"=100.0, "sampling info"=w776, "signal type"=T11."Square Wave", "phase"=0.0, "amplitude"=0.0, "frequency"=10.0) -> ("signal out"=w738:waveform(dbl))  [unwired: 2 in, 2 out]
        n170 = property on="Z-galvo Offset B slider" class="Slide (strict)"() -> ("Value"=w683:dbl)  [unwired: 2 in, 2 out]
        n171 = call-poly <vilib>:"DAQmx Timing.vi"("task/channels in"=w775, "sample mode"=w726, "waveform"=w727, "error in"=w774) -> ("task out"=w725:refnum<k21>, "error out"=w724:errorcluster)  [unwired: 10 in]
        n172 = property on="Z-Galvo Offset B (V)" class="DigNum (strict)"() -> ("Value"=w680:dbl)  [unwired: 2 in, 2 out]
        n173 = Multiply(x=w683, y=0.001) -> (x*y=w679:dbl)
        n174 = Add(x=w679, y=w680) -> (x+y=w681:dbl)
        n175 = First Call?() -> (First Call?: T/F=w757:bool)
        n176 = Select(t=w681, s=w696, f=0.0) -> (s? t:f=w698:dbl)
        n177 = call <vilib>:"Basic Function Generator.vi"("offset"=w698, "square wave duty cycle (%)"=100.0, "sampling info"=w776, "signal type"=T11."Square Wave", "phase"=0.0, "amplitude"=0.0, "frequency"=10.0) -> ("signal out"=w741:waveform(dbl))  [unwired: 2 in, 2 out]
        n178 = property on="Y-Galvo Offset B (V)" class="DigNum (strict)"() -> ("Value"=w706:dbl)  [unwired: 2 in, 2 out]
        n179 = Select(t=w692, s=w689, f=0.0) -> (s? t:f=w693:dbl)
        n180 = call <vilib>:"Basic Function Generator.vi"("offset"=w706, "sampling info"=w776, "signal type"=T11."Triangle Wave", "phase"=0.0, "amplitude"=w693, "frequency"=100.0) -> ("signal out"=w732:waveform(dbl))  [unwired: 3 in, 2 out]
        n181 = local read "Imaging Piezo Offset (V)\n(SPIM ARM A)"() -> (w710:dbl)
        n182 = call <vilib>:"Basic Function Generator.vi"("offset"=w710, "square wave duty cycle (%)"=100.0, "sampling info"=w776, "signal type"=T11."Square Wave", "phase"=0.0, "amplitude"=0.0, "frequency"=10.0) -> ("signal out"=w737:waveform(dbl))  [unwired: 2 in, 2 out]
        n183 = Build Array(w727, w764, w741, w732, w738, w737) -> (w748:waveform(dbl)[])
        n184 = call-poly <vilib>:"DAQmx Write.vi"("task/channels in"=w763, "data"=w748, "error in"=w762) -> ("task out"=w756:refnum<k21>, "error out"=w755:errorcluster)  [unwired: 10 in, 1 out]
        n185 = case shown="False" w757 {
          tunnel: [w797 w801] -> w779
          tunnel: [w796 w800] -> w778
          tunnel: w756 -> [w797 w799]
          tunnel: w755 -> [w796 w798]
          frame False {
          }
          frame True {
            n186 = call <vilib>:"DAQmx Start Task.vi"("task/channels in"=w799, "error in"=w798) -> ("task out"=w801:refnum<k21>, "error out"=w800:errorcluster)  [unwired: 12 in]
          }
        }
        n187 = First Call?() -> (First Call?: T/F=w719:bool)
        n188 = property on="Laser power (488 nm)" class="Slide (strict)"() -> ("Value"=w708:dbl)  [unwired: 2 in, 2 out]
        n189 = call <vilib>:"Basic Function Generator.vi"("offset"=w708, "sampling info"=w776, "amplitude"=0.0, "frequency"=10.0) -> ("signal out"=w722:waveform(dbl))  [unwired: 5 in, 2 out]
        n190 = property on="Laser power (561 nm)" class="Slide (strict)"() -> ("Value"=w707:dbl)  [unwired: 2 in, 2 out]
        n191 = call <vilib>:"Basic Function Generator.vi"("offset"=w707, "sampling info"=w776, "amplitude"=0.0, "frequency"=10.0) -> ("signal out"=w721:waveform(dbl))  [unwired: 5 in, 2 out]
        n192 = Divide(x=6.0 ("offset"), y=1.0) -> (x/y=w713:dbl)
        n193 = call <vilib>:"Basic Function Generator.vi"("offset"=w713, "sampling info"=w776, "signal type"=T11."Sine Wave", "amplitude"=0.0, "frequency"=10.0) -> ("signal out"=w711:waveform(dbl))  [unwired: 4 in, 2 out]
        n194 = Build Array(w722, w721, w711) -> (w720:waveform(dbl)[])
        n195 = call-poly <vilib>:"DAQmx Write.vi"("task/channels in"=w725, "data"=w720, "error in"=w724) -> ("task out"=w718:refnum<k21>, "error out"=w717:errorcluster)  [unwired: 10 in, 1 out]
        n196 = case shown="True" w719 {
          tunnel: [w791 w795] -> w771
          tunnel: [w790 w794] -> w770
          tunnel: w718 -> [w791 w793]
          tunnel: w717 -> [w790 w792]
          frame False {
          }
          frame True {
            n197 = call <vilib>:"DAQmx Start Task.vi"("task/channels in"=w793, "error in"=w792) -> ("task out"=w795:refnum<k21>, "error out"=w794:errorcluster)  [unwired: 12 in]
          }
        }
        n198 = Unbundle By Name(w711) -> ("t0"=w773:timestamp, "dt"=w772:dbl)  [unwired: 1 out]
        n199 = property on="Stop Adjustment" class="Bool (strict)"() -> ("Value"=w703:bool)  [unwired: 2 in, 2 out]
      }
      n200 = while {
        tunnel: w156 -> [w201]
        tunnel: [w202] -> w157
        stop <- w199 stop-if-true
        n201 = event shown="[3] \"Raise obj  bool\": Value Change" {
          selector: _ -> [_ _ _ _ _ _ _ _ _ _ _]
          dyn-events: _ -> [_ _ _ _ _ _ _ _ _ _ _]
          timeout: -1 -> [_ _ _ _ _ _ _ _ _ _ _]
          tunnel: w201 -> [w203 w206 w227 w250 w272 w293 w315 w335 w354 w373 w391]
          tunnel: [w203 w204 w226 w249 w271 w292 w314 w334 w353 w372 w391] -> w202
          tunnel: [_ _ _ _ _ _ _ _ _ _ TRUE] -> w199
          event Timeout {
            n202 = event-data() -> ()  [unwired: 1 in, 3 out]
          }
          event "Lower button": Value Change {
            # "Check the reply"
            # "Send the command"
            n203 = event-data() -> ()  [unwired: 1 in, 6 out]
            n204 = call-poly "VISA Configure Serial Port"("VISA resource name"=refnum<visa-resource-name> "COM6", "termination char\n(0xA = '\\n' = LF)"=u8 13 ("termination char\n(0xA = '\\n' = LF)"), "baud rate (9600)"=u32 115200, "error in (no error)"=w206) -> ("VISA resource name out"=w220:refnum<visa-resource-name>, "error out"=w219:errorcluster)  [unwired: 3 in, 7 out]
            n205 = property on="lower by" class="DigNum (strict)"() -> ("Value"=w205:dbl)  [unwired: 2 in, 2 out]
            n206 = VISA Flush I/O Buffer(VISA resource name=w220, mask (16)=u16 192 ("Mask"), error in (no error)=w219) -> (VISA resource name out=w217:refnum<visa-resource-name>, error out=w216:errorcluster)
            n207 = Multiply(x=w205, y=10.0) -> (x*y=w208:dbl)
            n208 = Format Into String(format string="R F=-%d" ("write buffer"), w208) -> (resulting string=w207:string)  [unwired: 2 in, 1 out]
            n209 = Concatenate Strings(w207, "\r\n") -> (w225:string)
            n210 = VISA Write(VISA resource name=w217, write buffer=w225, error in (no error)=w216) -> (VISA resource name out=w214:refnum<visa-resource-name>, error out=w213:errorcluster)  [unwired: 1 out]
            n211 = VISA Read "VISA Read 1"(VISA resource name=w214, byte count=u32 256, error in (no error)=w213) -> (VISA resource name out=w212:refnum<visa-resource-name>, error out=w211:errorcluster)  [unwired: 2 out]
            n212 = VISA Close(VISA resource name=w212, error in (no error)=w211) -> (error out=w204:errorcluster)
          }
          event "Raise button": Value Change {
            # "Check the reply"
            # "Send the command"
            n213 = event-data() -> ()  [unwired: 1 in, 6 out]
            n214 = property on="raise by" class="DigNum (strict)"() -> ("Value"=w247:dbl)  [unwired: 2 in, 2 out]
            n215 = call-poly "VISA Configure Serial Port"("VISA resource name"=refnum<visa-resource-name> "COM6", "termination char\n(0xA = '\\n' = LF)"=u8 13 ("termination char\n(0xA = '\\n' = LF)"), "baud rate (9600)"=u32 115200, "error in (no error)"=w227) -> ("VISA resource name out"=w241:refnum<visa-resource-name>, "error out"=w240:errorcluster)  [unwired: 3 in, 7 out]
            n216 = VISA Flush I/O Buffer(VISA resource name=w241, mask (16)=u16 192 ("Mask"), error in (no error)=w240) -> (VISA resource name out=w238:refnum<visa-resource-name>, error out=w237:errorcluster)
            n217 = Multiply(x=w247, y=10.0) -> (x*y=w229:dbl)
            n218 = Format Into String(format string="R F=%d" ("write buffer"), w229) -> (resulting string=w228:string)  [unwired: 2 in, 1 out]
            n219 = Concatenate Strings(w228, "\r\n") -> (w246:string)
            n220 = VISA Write(VISA resource name=w238, write buffer=w246, error in (no error)=w237) -> (VISA resource name out=w235:refnum<visa-resource-name>, error out=w234:errorcluster)  [unwired: 1 out]
            n221 = VISA Read "VISA Read 1"(VISA resource name=w235, byte count=u32 256, error in (no error)=w234) -> (VISA resource name out=w233:refnum<visa-resource-name>, error out=w232:errorcluster)  [unwired: 2 out]
            n222 = VISA Close(VISA resource name=w233, error in (no error)=w232) -> (error out=w226:errorcluster)
          }
          event "Raise obj \nbool": Value Change {
            # "Check the reply"
            # "Send the command"
            n223 = event-data() -> ()  [unwired: 1 in, 6 out]
            n224 = property on="Raise obj by" class="DigNum (strict)"() -> ("Value"=w248:dbl)  [unwired: 2 in, 2 out]
            n225 = call-poly "VISA Configure Serial Port"("VISA resource name"=refnum<visa-resource-name> "COM6", "termination char\n(0xA = '\\n' = LF)"=u8 13 ("termination char\n(0xA = '\\n' = LF)"), "baud rate (9600)"=u32 115200, "error in (no error)"=w250) -> ("VISA resource name out"=w256:refnum<visa-resource-name>, "error out"=w257:errorcluster)  [unwired: 3 in, 7 out]
            n226 = VISA Flush I/O Buffer(VISA resource name=w256, mask (16)=u16 192 ("Mask"), error in (no error)=w257) -> (VISA resource name out=w259:refnum<visa-resource-name>, error out=w260:errorcluster)
            n227 = Multiply(x=w248, y=10.0) -> (x*y=w268:dbl)
            n228 = Format Into String(format string="R Z=%d" ("write buffer"), w268) -> (resulting string=w269:string)  [unwired: 2 in, 1 out]
            n229 = Concatenate Strings(w269, "\r\n") -> (w251:string)
            n230 = VISA Write(VISA resource name=w259, write buffer=w251, error in (no error)=w260) -> (VISA resource name out=w262:refnum<visa-resource-name>, error out=w263:errorcluster)  [unwired: 1 out]
            n231 = VISA Read "VISA Read 1"(VISA resource name=w262, byte count=u32 256, error in (no error)=w263) -> (VISA resource name out=w264:refnum<visa-resource-name>, error out=w265:errorcluster)  [unwired: 2 out]
            n232 = VISA Close(VISA resource name=w264, error in (no error)=w265) -> (error out=w249:errorcluster)
          }
          event "Lower obj \nbool": Value Change {
            # "Check the reply"
            # "Send the command"
            n233 = event-data() -> ()  [unwired: 1 in, 6 out]
            n234 = property on="Lower obj by" class="DigNum (strict)"() -> ("Value"=w270:dbl)  [unwired: 2 in, 2 out]
            n235 = call-poly "VISA Configure Serial Port"("VISA resource name"=refnum<visa-resource-name> "COM6", "termination char\n(0xA = '\\n' = LF)"=u8 13 ("termination char\n(0xA = '\\n' = LF)"), "baud rate (9600)"=u32 115200, "error in (no error)"=w272) -> ("VISA resource name out"=w278:refnum<visa-resource-name>, "error out"=w279:errorcluster)  [unwired: 3 in, 7 out]
            n236 = VISA Flush I/O Buffer(VISA resource name=w278, mask (16)=u16 192 ("Mask"), error in (no error)=w279) -> (VISA resource name out=w281:refnum<visa-resource-name>, error out=w282:errorcluster)
            n237 = Multiply(x=w270, y=10.0) -> (x*y=w290:dbl)
            n238 = Format Into String(format string="R Z=-%d" ("write buffer"), w290) -> (resulting string=w291:string)  [unwired: 2 in, 1 out]
            n239 = Concatenate Strings(w291, "\r\n") -> (w273:string)
            n240 = VISA Write(VISA resource name=w281, write buffer=w273, error in (no error)=w282) -> (VISA resource name out=w284:refnum<visa-resource-name>, error out=w285:errorcluster)  [unwired: 1 out]
            n241 = VISA Read "VISA Read 1"(VISA resource name=w284, byte count=u32 256, error in (no error)=w285) -> (VISA resource name out=w286:refnum<visa-resource-name>, error out=w287:errorcluster)  [unwired: 2 out]
            n242 = VISA Close(VISA resource name=w286, error in (no error)=w287) -> (error out=w271:errorcluster)
          }
          event "Raise head to 25 mm": Value Change {
            # "Check the reply"
            # "Send the command"
            n243 = event-data() -> ()  [unwired: 1 in, 6 out]
            n244 = call-poly "VISA Configure Serial Port"("VISA resource name"=refnum<visa-resource-name> "COM6", "termination char\n(0xA = '\\n' = LF)"=u8 13 ("termination char\n(0xA = '\\n' = LF)"), "baud rate (9600)"=u32 115200, "error in (no error)"=w293) -> ("VISA resource name out"=w307:refnum<visa-resource-name>, "error out"=w306:errorcluster)  [unwired: 3 in, 7 out]
            n245 = VISA Flush I/O Buffer(VISA resource name=w307, mask (16)=u16 192 ("Mask"), error in (no error)=w306) -> (VISA resource name out=w304:refnum<visa-resource-name>, error out=w303:errorcluster)
            n246 = Multiply(x=25.0, y=10000.0) -> (x*y=w295:dbl)
            n247 = Format Into String(format string="MOVE F=%d" ("write buffer"), w295) -> (resulting string=w294:string)  [unwired: 2 in, 1 out]
            n248 = Concatenate Strings(w294, "\r\n") -> (w312:string)
            n249 = VISA Write(VISA resource name=w304, write buffer=w312, error in (no error)=w303) -> (VISA resource name out=w301:refnum<visa-resource-name>, error out=w300:errorcluster)  [unwired: 1 out]
            n250 = VISA Read "VISA Read 1"(VISA resource name=w301, byte count=u32 256, error in (no error)=w300) -> (VISA resource name out=w299:refnum<visa-resource-name>, error out=w298:errorcluster)  [unwired: 2 out]
            n251 = VISA Close(VISA resource name=w299, error in (no error)=w298) -> (error out=w292:errorcluster)
          }
          event "Lower head  to 1 mm": Value Change {
            # "Check the reply"
            # "Send the command"
            n252 = event-data() -> ()  [unwired: 1 in, 6 out]
            n253 = call-poly "VISA Configure Serial Port"("VISA resource name"=refnum<visa-resource-name> "COM6", "termination char\n(0xA = '\\n' = LF)"=u8 13 ("termination char\n(0xA = '\\n' = LF)"), "baud rate (9600)"=u32 115200, "error in (no error)"=w315) -> ("VISA resource name out"=w327:refnum<visa-resource-name>, "error out"=w326:errorcluster)  [unwired: 3 in, 7 out]
            n254 = VISA Flush I/O Buffer(VISA resource name=w327, mask (16)=u16 192 ("Mask"), error in (no error)=w326) -> (VISA resource name out=w324:refnum<visa-resource-name>, error out=w323:errorcluster)
            n255 = Format Into String(format string="MOVE F=%d" ("write buffer"), 10000.0 ("input 1")) -> (resulting string=w316:string)  [unwired: 2 in, 1 out]
            n256 = Concatenate Strings(w316, "\r\n") -> (w332:string)
            n257 = VISA Write(VISA resource name=w324, write buffer=w332, error in (no error)=w323) -> (VISA resource name out=w321:refnum<visa-resource-name>, error out=w320:errorcluster)  [unwired: 1 out]
            n258 = VISA Read "VISA Read 1"(VISA resource name=w321, byte count=u32 256, error in (no error)=w320) -> (VISA resource name out=w319:refnum<visa-resource-name>, error out=w318:errorcluster)  [unwired: 2 out]
            n259 = VISA Close(VISA resource name=w319, error in (no error)=w318) -> (error out=w314:errorcluster)
          }
          event "Halt": Value Change {
            # "Check the reply"
            # "Send the command"
            n260 = event-data() -> ()  [unwired: 1 in, 6 out]
            n261 = call-poly "VISA Configure Serial Port"("VISA resource name"=refnum<visa-resource-name> "COM6", "termination char\n(0xA = '\\n' = LF)"=u8 13 ("termination char\n(0xA = '\\n' = LF)"), "baud rate (9600)"=u32 115200, "error in (no error)"=w335) -> ("VISA resource name out"=w345:refnum<visa-resource-name>, "error out"=w344:errorcluster)  [unwired: 3 in, 7 out]
            n262 = VISA Flush I/O Buffer(VISA resource name=w345, mask (16)=u16 192 ("Mask"), error in (no error)=w344) -> (VISA resource name out=w342:refnum<visa-resource-name>, error out=w341:errorcluster)
            n263 = Concatenate Strings("HALT" ("write buffer"), "\r\n") -> (w351:string)
            n264 = VISA Write(VISA resource name=w342, write buffer=w351, error in (no error)=w341) -> (VISA resource name out=w339:refnum<visa-resource-name>, error out=w338:errorcluster)  [unwired: 1 out]
            n265 = VISA Read "VISA Read 1"(VISA resource name=w339, byte count=u32 256, error in (no error)=w338) -> (VISA resource name out=w337:refnum<visa-resource-name>, error out=w336:errorcluster)  [unwired: 2 out]
            n266 = VISA Close(VISA resource name=w337, error in (no error)=w336) -> (error out=w334:errorcluster)
          }
          event "LED power": Value Change {
            # "Check the reply"
            # "Send the command"
            n267 = event-data() -> ()  [unwired: 1 in, 6 out]
            n268 = call-poly "VISA Configure Serial Port"("VISA resource name"=refnum<visa-resource-name> "COM6", "termination char\n(0xA = '\\n' = LF)"=u8 13 ("termination char\n(0xA = '\\n' = LF)"), "baud rate (9600)"=u32 115200, "error in (no error)"=w354) -> ("VISA resource name out"=w360:refnum<visa-resource-name>, "error out"=w361:errorcluster)  [unwired: 3 in, 7 out]
            n269 = VISA Flush I/O Buffer(VISA resource name=w360, mask (16)=u16 192 ("Mask"), error in (no error)=w361) -> (VISA resource name out=w363:refnum<visa-resource-name>, error out=w364:errorcluster)
            n270 = property on="LED power" class="Slide (strict)"() -> ("Value"=w352:i32)  [unwired: 2 in, 2 out]
            n271 = Format Into String(format string="1LED X=%d" ("write buffer"), w352) -> (resulting string=w371:string)  [unwired: 2 in, 1 out]
            n272 = Concatenate Strings(w371, "\r\n") -> (w355:string)
            n273 = VISA Write(VISA resource name=w363, write buffer=w355, error in (no error)=w364) -> (VISA resource name out=w366:refnum<visa-resource-name>, error out=w367:errorcluster)  [unwired: 1 out]
            n274 = VISA Read "VISA Read 1"(VISA resource name=w366, byte count=u32 256, error in (no error)=w367) -> (VISA resource name out=w368:refnum<visa-resource-name>, error out=w369:errorcluster)  [unwired: 2 out]
            n275 = VISA Close(VISA resource name=w368, error in (no error)=w369) -> (error out=w353:errorcluster)
          }
          event "Switch to internal": Value Change {
            # "Check the reply"
            # "Send the command"
            n276 = event-data() -> ()  [unwired: 1 in, 6 out]
            n277 = call-poly "VISA Configure Serial Port"("VISA resource name"=refnum<visa-resource-name> "COM6", "termination char\n(0xA = '\\n' = LF)"=u8 13 ("termination char\n(0xA = '\\n' = LF)"), "baud rate (9600)"=u32 115200, "error in (no error)"=w373) -> ("VISA resource name out"=w384:refnum<visa-resource-name>, "error out"=w383:errorcluster)  [unwired: 3 in, 7 out]
            n278 = VISA Flush I/O Buffer(VISA resource name=w384, mask (16)=u16 192 ("Mask"), error in (no error)=w383) -> (VISA resource name out=w381:refnum<visa-resource-name>, error out=w380:errorcluster)
            n279 = Concatenate Strings("PM A=0 B=0 C=0 D=0 P=0 Q=0" ("write buffer"), "\r\n") -> (w389:string)
            n280 = VISA Write(VISA resource name=w381, write buffer=w389, error in (no error)=w380) -> (VISA resource name out=w378:refnum<visa-resource-name>, error out=w377:errorcluster)  [unwired: 1 out]
            n281 = VISA Read "VISA Read 1"(VISA resource name=w378, byte count=u32 256, error in (no error)=w377) -> (VISA resource name out=w376:refnum<visa-resource-name>, error out=w375:errorcluster)  [unwired: 2 out]
            n282 = property on="Scanner/Piezo \ncontrol mode" class="Str"("Value"="Switched to Internal (Tiger controller)" ("Scanner/Piezo control mode")) -> ()  [unwired: 2 in, 2 out]
            n283 = VISA Close(VISA resource name=w376, error in (no error)=w375) -> (error out=w372:errorcluster)
          }
          event "Stop Adjustment": Value Change {
            n284 = event-data() -> ()  [unwired: 1 in, 6 out]
          }
        }
        n285 = Wait (ms)(milliseconds to wait=u32 100) -> ()  [unwired: 1 out]
      }
      n286 = call "IMAQ Dispose"("Image"=w132, "error in (no error)"=w131) -> ("error out"=w130:errorcluster)  [unwired: 4 in]
      n287 = call "IMAQ Dispose"("Image"=w106, "error in (no error)"=w108) -> ("error out"=w107:errorcluster)  [unwired: 4 in]
      n288 = call "IMAQ Dispose"("Image"=w129, "error in (no error)"=w128) -> ("error out"=w127:errorcluster)  [unwired: 4 in]
      n289 = call <userlib>:"tm_stopcapture_40.vi"("error in (no error)"=w127, "Handle in"=w133) -> ("error out"=w138:errorcluster, "Handle out"=w137:u32)  [unwired: 8 in]
      n290 = call <userlib>:"tm_stopcapture_40.vi"("error in (no error)"=w107, "Handle in"=w112) -> ("error out"=w117:errorcluster, "Handle out"=w116:u32)  [unwired: 8 in]
      n291 = call <userlib>:"LuStopStream.vi"("error in"=w130, "handle in"=w146) -> ("error out"=w147:errorcluster, "Handle out"=w148:u64)  [unwired: 8 in]
      n292 = call <userlib>:"tm_unpreparecapture_40.vi"("error in (no error)"=w117, "Handle in"=w116) -> ("error out"=w115:errorcluster, "Handle out"=w114:u32)  [unwired: 8 in]
      n293 = call <userlib>:"LuCameraClose.vi"("error in (no error)"=w147, "Camera handle in"=w148) -> ("error out"=w145:errorcluster)  [unwired: 7 in]
      n294 = call <userlib>:"tm_unpreparecapture_40.vi"("error in (no error)"=w138, "Handle in"=w137) -> ("error out"=w136:errorcluster, "Handle out"=w135:u32)  [unwired: 8 in]
      n295 = call <userlib>:"tm_closecamera_40.vi"("error in (no error)"=w115, "Handle in"=w114) -> ("error out"=w113:errorcluster)  [unwired: 9 in]
      n296 = call <userlib>:"tm_closecamera_40.vi"("error in (no error)"=w136, "Handle in"=w135) -> ("error out"=w134:errorcluster)  [unwired: 9 in]
      n297 = call <userlib>:"tm_deinitialize_40.vi"("error in (no error)"=w113) -> ("error out"=w110:errorcluster)  [unwired: 10 in]
      n298 = call <userlib>:"tm_deinitialize_40.vi"("error in (no error)"=w134) -> ("error out"=w111:errorcluster)  [unwired: 10 in]
      n299 = call <vilib>:"DAQmx Clear Task.vi"("task in"=w191, "error in"=w190) -> ("error out"=→"DAQ1 error (adjustment)":errorcluster)  [unwired: 13 in]
      n300 = call <vilib>:"DAQmx Stop Task.vi"("task/channels in"=w165, "error in"=w164) -> ("task out"=w163:refnum<k21>, "error out"=w162:errorcluster)  [unwired: 12 in]
      n301 = Initialize Array(0.0 ("element"), 100 ("dimension size")) -> (w174:dbl[])
      n302 = Bundle By Name("Y"=w174, "t0"=w176, "dt"=w175) -> (w171:waveform(dbl))  [unwired: 1 in]
      n303 = Merge Errors(w111, w110) -> (w109:errorcluster)
      n304 = Build Array(w171, w171, w171) -> (w170:waveform(dbl)[])
      n305 = call-poly <vilib>:"DAQmx Write.vi"("task/channels in"=w163, "data"=w170, "error in"=w162) -> ("task out"=w169:refnum<k21>, "error out"=w168:errorcluster)  [unwired: 10 in, 1 out]
      n306 = call <vilib>:"DAQmx Start Task.vi"("task/channels in"=w169, "error in"=w168) -> ("task out"=w167:refnum<k21>, "error out"=w166:errorcluster)  [unwired: 12 in]
      n307 = call <vilib>:"DAQmx Clear Task.vi"("task in"=w167, "error in"=w166) -> ("error out"=→"DAQ2 error (adjustment)":errorcluster)  [unwired: 13 in]
    }
    frame "Image Acquisition - Single Color" {
      n308 = call <userlib>:"tm_initialize_40.vi"() -> ("error out"=w865:errorcluster, "Number Of Cameras"=w864:u32)  [unwired: 8 in, 2 out]
      n309 = call "get_stage_loc.vi"("error in (no error)"=w812) -> ("String"=w806:string)  [unwired: 10 in]
      n310 = Build Path(base path=w811, name or relative path=w810) -> (appended path=w807:path)
      n311 = Not Equal To 0?(x=w864) -> ()  [unwired: 1 out]
      n312 = Build Path(base path=w807, name or relative path="Imaging  Conditions.txt") -> (appended path=w808:path)
      n313 = call "MakeImagCondFileContents.vi"("Cluster"=w805, "Position"=w806, "StorageDirPath"=w807) -> ("StringOutToFile"=w804:string)  [unwired: 8 in]
      n314 = flat-sequence {
        tunnel: w865 -> [w880]
        tunnel: w863 -> [w879]
        tunnel: w862 -> [w878]
        tunnel: [w875] -> w840
        tunnel: [w874] -> w838
        tunnel: [w877] -> w836
        tunnel: [w876] -> w834
        tunnel: [w870] -> w832
        tunnel: [w866] -> w802
        tunnel: w840 -> [w889]
        tunnel: [w886] -> w839
        tunnel: w838 -> [w887]
        tunnel: [w892] -> w837
        tunnel: w836 -> [w888]
        tunnel: [w891] -> w835
        tunnel: w834 -> [w890]
        tunnel: [w885] -> w833
        tunnel: w832 -> [w897]
        tunnel: [w897] -> w831
        tunnel: [w896] -> w830
        tunnel: [w895] -> w829
        tunnel: w828 -> [w894]
        tunnel: w827 -> [w893]
        tunnel: w826 -> [w884]
        tunnel: w802 -> [w883]
        tunnel: w861 -> [w955]
        tunnel: w860 -> [w954]
        tunnel: w839 -> [w963]
        tunnel: w837 -> [w949]
        tunnel: w835 -> [w948]
        tunnel: w833 -> [w962]
        tunnel: [w961] -> w859
        tunnel: [w956] -> w858
        tunnel: [w960] -> w825
        tunnel: [w959] -> w823
        tunnel: [w958] -> w821
        tunnel: [w957] -> w819
        tunnel: w826 -> [w947]
        tunnel: w831 -> [w952]
        tunnel: w830 -> [w951]
        tunnel: w829 -> [w950]
        tunnel: w825 -> [w1011]
        tunnel: [w1011] -> w824
        tunnel: w823 -> [w1010]
        tunnel: [w1010] -> w822
        tunnel: w821 -> [w1009]
        tunnel: [w1009] -> w820
        tunnel: w819 -> [w1008]
        tunnel: [w1008] -> w818
        tunnel: [w1007] -> w817
        tunnel: w816 -> [w1003]
        tunnel: w815 -> [w1002]
        tunnel: w814 -> [w1001]
        tunnel: w813 -> [w1000]
        tunnel: w824 -> [w1064]
        tunnel: w822 -> [w1066]
        tunnel: w820 -> [w1068]
        tunnel: w818 -> [w1071]
        tunnel: w850 -> [w1063]
        tunnel: w849 -> [w1062]
        tunnel: [w1065] -> w848
        tunnel: [w1069] -> w847
        tunnel: [w1070] -> w846
        tunnel: [w1067] -> w845
        tunnel: [w1061] -> w843
        tunnel: w842 -> [w1060]
        tunnel: w841 -> [w1059]
        tunnel: w817 -> [w1045]
        tunnel: [w1128] -> w851
        tunnel: [w1129] -> w854
        tunnel: [w1130] -> w853
        tunnel: [w1131] -> w852
        tunnel: w848 -> [w1131]
        tunnel: w847 -> [w1130]
        tunnel: w846 -> [w1129]
        tunnel: w845 -> [w1128]
        tunnel: w843 -> [w1126]
        frame #0 {
          n315 = local read "AutoFocus \n(move only piezo)"() -> (w868:bool)
          n316 = property on="Bgndbool" class="Bool (strict)"() -> ("Value"=w866:bool)  [unwired: 2 in, 2 out]
          n317 = property on="Autofocus \n(move only galvo )" class="Bool (strict)"() -> ("Value"=w869:bool)  [unwired: 2 in, 2 out]
          n318 = Or(x=w868, y=w869) -> (x .or. y?=w867:bool)
          n319 = property on="Force Cameras Open" class="Bool (strict)"() -> ("Value"=w871:bool)  [unwired: 2 in, 2 out]
          n320 = call "camera initialization.vi"("Camera SPIMB"=w878, "Force Open"=w871, "error in (no error)"=w880, "Camera SPIMA"=w879) -> ("SPIMB Out"=w874:u32, "SPIMB Error"=w875:errorcluster, "SPIMB Serial No"=w872:string, "SPIMA Out"=w877:u32, "SPIMA Error"=w876:errorcluster, "SPIMA Serial No"=w873:string)  [unwired: 10 in]
          n321 = case shown="False" w867 {
            tunnel: [w881 1] -> w870
            frame False {
              n322 = property on="# of Volumes" class="DigNum (strict)"() -> ("Value"=w881:dbl)  [unwired: 2 in, 2 out]
            }
            frame True {
            }
          }
          n323 = property on="Volume Indicator" class="Slide (strict)"("Scale.Maximum"=w870) -> ()  [unwired: 2 in, 2 out]
          n324 = property on="Camera A ID:" class="Str"("Value"=w873) -> ()  [unwired: 2 in, 2 out]
          n325 = property on="Camera B ID:" class="Str"("Value"=w872) -> ()  [unwired: 2 in, 2 out]
        }
        frame #1 {
          n326 = property on="Prefix for \nimage \nfilenames" class="Str"() -> ("Value"=w896:string)  [unwired: 2 in, 2 out]
          n327 = property on="Capture \nImages \nOn/Off" class="Bool (strict)"() -> ("Value"=w895:bool)  [unwired: 2 in, 2 out]
          n328 = case shown="True" w883 {
            tunnel: w896 -> [_ w924]
            tunnel: w895 -> [_ w921]
            tunnel: w894 -> [_ w920]
            tunnel: w893 -> [_ w919]
            tunnel: [w899 w918] -> w892
            tunnel: [w898 w917] -> w891
            tunnel: w890 -> [w900 w915]
            tunnel: w889 -> [w901 w914]
            tunnel: w888 -> [w899 w913]
            tunnel: w887 -> [w898 w912]
            tunnel: [w901 w911] -> w886
            tunnel: [w900 w910] -> w885
            tunnel: w884 -> [_ w908]
            frame False {
            }
            frame True {
              w907 = 0.0 ("Y-Gal ampl")
              n329 = Bundle(cluster=w908, "Y-Gal ampl"=w907, "A Z-Gal amp"=w907, "A Z-Gal Off"=w907, "B Z-Gal Amp"=w907, "B Z-Gal Off"=w907, "A Y-Gal Off"=w907, "B Y-Gal Off"=w907) -> (w904:T9)  [unwired: 9 in]
              n330 = Concatenate Strings(w924, "_bgnd" ("string")) -> (w922:string)
              n331 = call "Stage_1_waveform_for_DAQ.vi"("input cluster"=w904) -> ("DAQ cluster"=w905:T17, "Time cluster"=w906:cluster{"Total time":dbl, "Time per step":dbl})  [unwired: 9 in]
              n332 = call "Stage_2_waveform_for_DAQ.vi"("input cluster"=w904) -> ("DAQ cluster"=w902:T17, "time cluster"=w903:cluster{"total time":dbl, "time per step":dbl})  [unwired: 9 in]
              n333 = for {
                N: 5 -> [_]
                tunnel: w922 -> [w942]
                tunnel: w921 -> [w941]
                tunnel: w920 -> [w940]
                tunnel: w919 -> [w939]
                tunnel: w913 -> [w938]
                tunnel: [w937] -> w918
                tunnel: [w936] -> w917
                tunnel: w915 -> [w935]
                tunnel: w914 -> [w934]
                tunnel: w912 -> [w932]
                tunnel: [w931] -> w911
                tunnel: [w930] -> w910
                tunnel: w904 -> [w929]
                tunnel: w906 -> [w928]
                tunnel: w905 -> [w927]
                tunnel: w903 -> [w926]
                tunnel: w902 -> [w925]
                i -> [w933]
                n334 = call "capture_single_color_dual_view (SubVI).vi"("SpimA path"=w940, "Control values"=w929, "volume number"=w933, "filename prefix"=w942, "Cam A handle in"=w938, "Capture on/off"=w941, "Cam A error in"=w935, "Cam B error in"=w934, "SpimB path"=w939, "Stage 1 time cluster"=w928, "Cam B handle in"=w932, "Stage 1 DAQ cluster"=w927, "Stage 2 time cluster"=w926, "stage 2 DAQ cluster"=w925) -> ("Camera A error out"=w930:errorcluster, "Camera A handle"=w937:u32, "Camera B handle"=w936:u32, "Camera B error out"=w931:errorcluster)  [unwired: 1 in, 9 out]
              }
              n335 = property on="Acquisition status:" class="Str"("Value"="Acquiring background..." ("Acquisition status:")) -> ()  [unwired: 2 in, 2 out]
            }
          }
        }
        frame #2 {
          n336 = call "Stage_1_waveform_for_DAQ.vi"("input cluster"=w947) -> ("DAQ cluster"=w945:T17, "Time cluster"=w946:cluster{"Total time":dbl, "Time per step":dbl})  [unwired: 9 in]
          n337 = call "Stage_2_waveform_for_DAQ.vi"("input cluster"=w947) -> ("DAQ cluster"=w943:T17, "time cluster"=w944:cluster{"total time":dbl, "time per step":dbl})  [unwired: 9 in]
          n338 = for {
            N: w952 -> [_]
            tunnel: w955 -> [w976]
            tunnel: w963 -> [w978]
            tunnel: w948 -> [w979]
            tunnel: w949 -> [w991]
            tunnel: w962 -> [w990]
            tunnel: [w989] -> w961
            tunnel: [w988] -> w960
            tunnel: [w987] -> w959
            tunnel: [w986] -> w958
            tunnel: [w985] -> w957
            tunnel: [w984] -> w956
            tunnel: w954 -> [w974]
            tunnel: w947 -> [w971]
            tunnel: w951 -> [w972]
            tunnel: w950 -> [w970]
            tunnel: w946 -> [w967]
            tunnel: w945 -> [w966]
            tunnel: w944 -> [w965]
            tunnel: w943 -> [w964]
            i -> [w973]
            n339 = call "capture_single_color_dual_view (SubVI).vi"("SpimA path"=w974, "Control values"=w971, "volume number"=w973, "filename prefix"=w972, "Cam A handle in"=w991, "Capture on/off"=w970, "Cam A error in"=w990, "Cam B error in"=w978, "SpimB path"=w976, "Stage 1 time cluster"=w967, "Cam B handle in"=w979, "Stage 1 DAQ cluster"=w966, "Stage 2 time cluster"=w965, "stage 2 DAQ cluster"=w964) -> ("Stage 0"=→"stage0":u32, "Stage 1"=→"stage1":u32, "Stage 2"=→"stage2":u32, "Stage 3"=→"stage 3":u32, "Cam B Frame Count"=w969:i32, "Camera A error out"=w986:errorcluster, "DAC card stage A error"=w984:errorcluster, "DAC card stage B error"=w989:errorcluster, "interstage"=→"interstage":u32, "Camera A handle"=w985:u32, "Camera B handle"=w987:u32, "Cam A Frame Count"=w968:i32, "Camera B error out"=w988:errorcluster)  [unwired: 1 in]
            n340 = property on="Time Point Delay" class="DigNum (strict)"() -> ("Value"=w975:dbl)  [unwired: 2 in, 2 out]
            n341 = Wait (ms)(milliseconds to wait=w975) -> ()  [unwired: 1 out]
            n342 = property on="Volume Indicator" class="Slide (strict)"("Value"=w973) -> ()  [unwired: 2 in, 2 out]
            n343 = property on="planes acquired (A)" class="DigNum (strict)"("Value"=w968) -> ()  [unwired: 2 in, 2 out]
            n344 = property on="planes acquired (B)" class="DigNum (strict)"("Value"=w969) -> ()  [unwired: 2 in, 2 out]
          }
          n345 = local write "Acquisition status:"("Acquiring images..." ("Program status")) -> ()
        }
        frame #3 {
          n346 = property on="Bgndbool" class="Bool (strict)"() -> ("Value"=w999:bool)  [unwired: 2 in, 2 out]
          n347 = property on="Capture Images On/Off" class="Bool (strict)"() -> ("Value"=w1005:bool)  [unwired: 2 in, 2 out]
          n348 = property on="Export to TIFF" class="Bool (strict)"() -> ("Value"=w1006:bool)  [unwired: 2 in, 2 out]
          n349 = property on="Prefix for image filenames" class="Str"() -> ("Value"=w998:string)  [unwired: 2 in, 2 out]
          n350 = Compound Arithmetic op=AND(w1006, w1005, w999) -> (w1004:bool)
          n351 = Concatenate Strings(w998, "_bgnd" ("string")) -> (w994:string)
          n352 = Concatenate Strings(w994, "_A" ("string")) -> (w993:string)
          n353 = Concatenate Strings(w994, "_B" ("string")) -> (w992:string)
          n354 = case shown="True" w1004 {
            tunnel: w1003 -> [_ w1021]
            tunnel: w1002 -> [_ w1020]
            tunnel: [w1012 w1019] -> w1007
            tunnel: w1001 -> [_ w1018]
            tunnel: w1000 -> [_ w1017]
            tunnel: w993 -> [_ w1016]
            tunnel: w992 -> [_ w1015]
            frame False {
              n355 = xnode "Error Ring"() -> ("error out"=w1012:errorcluster)
            }
            frame True {
              n356 = for {
                N: 5 -> [_]
                tunnel: w1021 -> [w1032]
                tunnel: w1020 -> [w1031]
                tunnel: [w1024] -> w1019
                tunnel: w1018 -> [w1030]
                tunnel: w1017 -> [w1029]
                tunnel: w1016 -> [w1023]
                tunnel: w1015 -> [w1022]
                i -> [w1028]
                n357 = flat-sequence {
                  tunnel: w1032 -> [w1038]
                  tunnel: w1028 -> [w1036]
                  tunnel: w1030 -> [w1037]
                  tunnel: [w1036] -> w1027
                  tunnel: [w1035] -> w1025
                  tunnel: w1023 -> [w1034]
                  tunnel: w1031 -> [w1044]
                  tunnel: w1029 -> [w1043]
                  tunnel: w1027 -> [w1042]
                  tunnel: [w1041] -> w1026
                  tunnel: w1022 -> [w1040]
                  frame #0 {
                    n358 = call "DCIMG to TIFF conversion_multiple files.vi"("Volume number"=w1036, "IsSingleColor"=TRUE, "Input File Path"=w1038, "Input File Name"=w1034, "Output Path"=w1037) -> ("Error Out"=w1035:errorcluster)  [unwired: 5 in, 5 out]
                  }
                  frame #1 {
                    n359 = call "DCIMG to TIFF conversion_multiple files.vi"("Volume number"=w1042, "IsSingleColor"=TRUE, "Input File Path"=w1044, "Input File Name"=w1040, "Output Path"=w1043) -> ("Error Out"=w1041:errorcluster)  [unwired: 5 in, 5 out]
                  }
                }
                n360 = Merge Errors(w1026, w1025) -> (w1024:errorcluster)
              }
            }
          }
        }
        frame #4 {
          n361 = property on="Export to\n TIFF" class="Bool (strict)"() -> ("Value"=w1053:bool)  [unwired: 2 in, 2 out]
          n362 = property on="Autofocus \n(move only galvo )" class="Bool (strict)"() -> ("Value"=w1046:bool)  [unwired: 2 in, 2 out]
          n363 = property on="AutoFocus \n(move only piezo)" class="Bool (strict)"() -> ("Value"=w1047:bool)  [unwired: 2 in, 2 out]
          n364 = property on="Capture\n Images \nOn/Off" class="Bool (strict)"() -> ("Value"=w1054:bool)  [unwired: 2 in, 2 out]
          n365 = And(x=w1053, y=w1054) -> (x .and. y?=w1052:bool)
          n366 = Or(x=w1047, y=w1046) -> (x .or. y?=w1048:bool)
          n367 = case shown="False" w1048 {
            tunnel: [w1073 1] -> w1049
            frame False {
              n368 = property on="# of \nVolumes" class="DigNum (strict)"() -> ("Value"=w1073:dbl)  [unwired: 2 in, 2 out]
            }
            frame True {
            }
          }
          n369 = property on="Prefix for image\n filenames" class="Str"() -> ("Value"=w1056:string)  [unwired: 2 in, 2 out]
          n370 = Concatenate Strings(w1056, "_A" ("string")) -> (w1051:string)
          n371 = Concatenate Strings(w1056, "_B" ("string")) -> (w1050:string)
          n372 = case shown="True" w1052 {
            tunnel: w1071 -> [w1079 w1097]
            tunnel: [w1079 w1096] -> w1070
            tunnel: [w1078 w1095] -> w1069
            tunnel: w1068 -> [w1078 w1094]
            tunnel: [w1077 w1093] -> w1067
            tunnel: w1066 -> [w1077 w1092]
            tunnel: [w1076 w1091] -> w1065
            tunnel: w1064 -> [w1076 w1090]
            tunnel: w1063 -> [_ w1089]
            tunnel: w1062 -> [_ w1088]
            tunnel: w1049 -> [_ w1087]
            tunnel: [w1075 w1086] -> w1061
            tunnel: w1060 -> [_ w1085]
            tunnel: w1059 -> [_ w1084]
            tunnel: w1051 -> [_ w1083]
            tunnel: w1050 -> [_ w1082]
            tunnel: w1045 -> [_ w1081]
            frame False {
              n373 = xnode "Error Ring"() -> ("error out"=w1075:errorcluster)
            }
            frame True {
              n374 = for {
                N: w1087 -> [_]
                tunnel: w1097 -> [w1113]
                tunnel: [w1113] -> w1096
                tunnel: [w1112] -> w1095
                tunnel: w1094 -> [w1112]
                tunnel: [w1111] -> w1093
                tunnel: w1092 -> [w1111]
                tunnel: [w1110] -> w1091
                tunnel: w1090 -> [w1110]
                tunnel: w1089 -> [w1109]
                tunnel: w1088 -> [w1108]
                tunnel: [w1101] -> w1086
                tunnel: w1085 -> [w1107]
                tunnel: w1084 -> [w1106]
                tunnel: w1083 -> [w1100]
                tunnel: w1082 -> [w1099]
                tunnel: w1081 -> [w1098]
                i -> [w1105]
                n375 = flat-sequence {
                  tunnel: w1109 -> [w1119]
                  tunnel: w1105 -> [w1117]
                  tunnel: w1107 -> [w1118]
                  tunnel: [w1117] -> w1104
                  tunnel: [w1116] -> w1102
                  tunnel: w1100 -> [w1115]
                  tunnel: w1108 -> [w1125]
                  tunnel: w1106 -> [w1124]
                  tunnel: w1104 -> [w1123]
                  tunnel: [w1122] -> w1103
                  tunnel: w1099 -> [w1121]
                  frame #0 {
                    n376 = call "DCIMG to TIFF conversion_multiple files.vi"("Volume number"=w1117, "IsSingleColor"=TRUE, "Input File Path"=w1119, "Input File Name"=w1115, "Output Path"=w1118) -> ("Error Out"=w1116:errorcluster)  [unwired: 5 in, 5 out]
                  }
                  frame #1 {
                    n377 = call "DCIMG to TIFF conversion_multiple files.vi"("Volume number"=w1123, "IsSingleColor"=TRUE, "Input File Path"=w1125, "Input File Name"=w1121, "Output Path"=w1124) -> ("Error Out"=w1122:errorcluster)  [unwired: 5 in, 5 out]
                  }
                }
                n378 = property on="Volume Indicator" class="Slide (strict)"("Value"=w1105) -> ()  [unwired: 2 in, 2 out]
                n379 = Merge Errors(w1103, w1102, w1098) -> (w1101:errorcluster)
              }
            }
          }
          n380 = local read "AutoFocus \n(move only piezo)"() -> (w1072:bool)
          n381 = local write "Acquisition status:"("Exporting DCIMG to TIFFs..." ("Program status")) -> ()
          n382 = case shown="True" w1072 {
            frame False {
            }
            frame True {
            }
          }
        }
        frame #5 {
          n383 = local write "Acquisition status:"("Done." ("Program status")) -> ()
          "File conversion error" <- w1126
        }
      }
      n384 = Write to Text File(file (use dialog)=w808, text=w804) -> (error out=w803:errorcluster)  [unwired: 2 in, 2 out]
      n385 = call <userlib>:"tm_closecamera_40.vi"("error in (no error)"=w852, "Handle in"=w851) -> ("error out"=w857:errorcluster)  [unwired: 9 in]
      n386 = call <userlib>:"tm_closecamera_40.vi"("error in (no error)"=w853, "Handle in"=w854) -> ("error out"=w856:errorcluster)  [unwired: 9 in]
      n387 = Merge Errors(w856, w857) -> (w855:errorcluster)
      n388 = call <userlib>:"tm_deinitialize_40.vi"("error in (no error)"=w855) -> ("error out"=w844:errorcluster)  [unwired: 10 in]
    }
    frame "Image Acquisition - Dual Color" {
      n389 = call "get_stage_loc.vi"("error in (no error)"=w1141) -> ("String"=w1136:string)  [unwired: 10 in]
      n390 = call <userlib>:"tm_initialize_40.vi"() -> ("error out"=w1143:errorcluster, "Number Of Cameras"=w1142:u32)  [unwired: 8 in, 2 out]
      n391 = Not Equal To 0?(x=w1142) -> ()  [unwired: 1 out]
      n392 = Build Path(base path=w1133, name or relative path=w1132) -> (appended path=w1138:path)
      n393 = flat-sequence {
        tunnel: w1143 -> [w1188]
        tunnel: w1176 -> [w1187]
        tunnel: w1175 -> [w1186]
        tunnel: [w1183] -> w1172
        tunnel: [w1182] -> w1171
        tunnel: [w1185] -> w1170
        tunnel: [w1184] -> w1169
        tunnel: [w1178] -> w1144
        tunnel: w1174 -> [w1197]
        tunnel: w1173 -> [w1196]
        tunnel: w1172 -> [w1207]
        tunnel: w1171 -> [w1206]
        tunnel: w1170 -> [w1205]
        tunnel: w1169 -> [w1204]
        tunnel: [w1203] -> w1168
        tunnel: [w1198] -> w1167
        tunnel: [w1202] -> w1160
        tunnel: [w1201] -> w1159
        tunnel: [w1200] -> w1158
        tunnel: [w1199] -> w1157
        tunnel: w1145 -> [w1194]
        tunnel: w1144 -> [w1193]
        tunnel: w1160 -> [w1248]
        tunnel: w1159 -> [w1250]
        tunnel: w1158 -> [w1252]
        tunnel: w1157 -> [w1255]
        tunnel: w1155 -> [w1247]
        tunnel: w1154 -> [w1246]
        tunnel: [w1249] -> w1153
        tunnel: [w1253] -> w1152
        tunnel: [w1254] -> w1151
        tunnel: [w1251] -> w1150
        tunnel: [w1245] -> w1148
        tunnel: w1147 -> [w1244]
        tunnel: w1146 -> [w1243]
        tunnel: [w1310] -> w1156
        tunnel: [w1311] -> w1163
        tunnel: [w1312] -> w1162
        tunnel: [w1313] -> w1161
        tunnel: w1153 -> [w1313]
        tunnel: w1152 -> [w1312]
        tunnel: w1151 -> [w1311]
        tunnel: w1150 -> [w1310]
        tunnel: w1148 -> [w1308]
        frame #0 {
          n394 = local read "AutoFocus \n(move only piezo)"() -> (w1177:bool)
          n395 = property on="Force Cameras Open" class="Bool (strict)"() -> ("Value"=w1179:bool)  [unwired: 2 in, 2 out]
          n396 = call "camera initialization.vi"("Camera SPIMB"=w1186, "Force Open"=w1179, "error in (no error)"=w1188, "Camera SPIMA"=w1187) -> ("SPIMB Out"=w1182:u32, "SPIMB Error"=w1183:errorcluster, "SPIMB Serial No"=w1180:string, "SPIMA Out"=w1185:u32, "SPIMA Error"=w1184:errorcluster, "SPIMA Serial No"=w1181:string)  [unwired: 10 in]
          n397 = case shown="False" w1177 {
            tunnel: [w1189 1] -> w1178
            frame False {
              n398 = property on="# of Volumes" class="DigNum (strict)"() -> ("Value"=w1189:dbl)  [unwired: 2 in, 2 out]
            }
            frame True {
            }
          }
          n399 = property on="Volume Indicator" class="Slide (strict)"("Scale.Maximum"=w1178) -> ()  [unwired: 2 in, 2 out]
          n400 = property on="Camera A ID:" class="Str"("Value"=w1181) -> ()  [unwired: 2 in, 2 out]
          n401 = property on="Camera B ID:" class="Str"("Value"=w1180) -> ()  [unwired: 2 in, 2 out]
        }
        frame #1 {
          n402 = property on="Prefix for \nimage \nfilenames" class="Str"() -> ("Value"=w1192:string)  [unwired: 2 in, 2 out]
          n403 = property on="Capture \nImages \nOn/Off" class="Bool (strict)"() -> ("Value"=w1191:bool)  [unwired: 2 in, 2 out]
          n404 = for {
            N: w1193 -> [_]
            tunnel: w1197 -> [w1216]
            tunnel: w1207 -> [w1218]
            tunnel: w1206 -> [w1219]
            tunnel: w1205 -> [w1231]
            tunnel: w1204 -> [w1230]
            tunnel: [w1229] -> w1203
            tunnel: [w1228] -> w1202
            tunnel: [w1227] -> w1201
            tunnel: [w1226] -> w1200
            tunnel: [w1225] -> w1199
            tunnel: [w1224] -> w1198
            tunnel: w1196 -> [w1214]
            tunnel: w1194 -> [w1211]
            tunnel: w1192 -> [w1212]
            tunnel: w1191 -> [w1210]
            i -> [w1213]
            n405 = property on="Time Point Delay" class="DigNum (strict)"() -> ("Value"=w1215:dbl)  [unwired: 2 in, 2 out]
            n406 = Wait (ms)(milliseconds to wait=w1215) -> ()  [unwired: 1 out]
            n407 = property on="Volume Indicator" class="Slide (strict)"("Value"=w1213) -> ()  [unwired: 2 in, 2 out]
            n408 = call "capture_dual_color_dual_view (SubVI).vi"("SpimA path"=w1214, "Control values"=w1211, "volume number"=w1213, "filename prefix"=w1212, "Cam A handle in"=w1231, "Capture on/off"=w1210, "Cam A error in"=w1230, "Cam B error in"=w1218, "SpimB path"=w1216, "Cam B handle in"=w1219) -> ("Stage 0"=→"stage0 2":u32, "Stage 1"=→"stage1 2":u32, "Stage 2"=→"stage2 2":u32, "Stage 3"=→"stage 4":u32, "Cam B Frame Count"=w1209:i32, "Camera A error out"=w1226:errorcluster, "DAC card stage A error"=w1224:errorcluster, "DAC card stage B error"=w1229:errorcluster, "interstage"=→"interstage 2":u32, "Camera A handle"=w1225:u32, "Camera B handle"=w1227:u32, "Cam A Frame Count"=w1208:i32, "Camera B error out"=w1228:errorcluster)  [unwired: 5 in]
            n409 = property on="planes acquired (A)" class="DigNum (strict)"("Value"=w1208) -> ()  [unwired: 2 in, 2 out]
            n410 = property on="planes acquired (B)" class="DigNum (strict)"("Value"=w1209) -> ()  [unwired: 2 in, 2 out]
          }
          n411 = local write "Acquisition status:"("Acquiring images..." ("Program status")) -> ()
        }
        frame #2 {
          n412 = property on="AutoFocus \n(move only piezo)" class="Bool (strict)"() -> ("Value"=w1232:bool)  [unwired: 2 in, 2 out]
          n413 = property on="Export to\n TIFF" class="Bool (strict)"() -> ("Value"=w1237:bool)  [unwired: 2 in, 2 out]
          n414 = property on="Capture\n Images \nOn/Off" class="Bool (strict)"() -> ("Value"=w1238:bool)  [unwired: 2 in, 2 out]
          n415 = case shown="False" w1232 {
            tunnel: [w1257 1] -> w1233
            frame False {
              n416 = property on="# of Volumes" class="DigNum (strict)"() -> ("Value"=w1257:dbl)  [unwired: 2 in, 2 out]
            }
            frame True {
            }
          }
          n417 = And(x=w1237, y=w1238) -> (x .and. y?=w1236:bool)
          n418 = property on="Prefix for image\n filenames" class="Str"() -> ("Value"=w1240:string)  [unwired: 2 in, 2 out]
          n419 = Concatenate Strings(w1240, "_A" ("string")) -> (w1235:string)
          n420 = Concatenate Strings(w1240, "_B" ("string")) -> (w1234:string)
          n421 = case shown="True" w1236 {
            tunnel: w1255 -> [w1263 w1280]
            tunnel: [w1263 w1279] -> w1254
            tunnel: [w1262 w1278] -> w1253
            tunnel: w1252 -> [w1262 w1277]
            tunnel: [w1261 w1276] -> w1251
            tunnel: w1250 -> [w1261 w1275]
            tunnel: [w1260 w1274] -> w1249
            tunnel: w1248 -> [w1260 w1273]
            tunnel: w1247 -> [_ w1272]
            tunnel: w1246 -> [_ w1271]
            tunnel: w1233 -> [_ w1270]
            tunnel: [w1259 w1269] -> w1245
            tunnel: w1244 -> [_ w1268]
            tunnel: w1243 -> [_ w1267]
            tunnel: w1235 -> [_ w1266]
            tunnel: w1234 -> [_ w1265]
            frame False {
              n422 = xnode "Error Ring"() -> ("error out"=w1259:errorcluster)
            }
            frame True {
              n423 = for {
                N: w1270 -> [_]
                tunnel: w1280 -> [w1295]
                tunnel: [w1295] -> w1279
                tunnel: [w1294] -> w1278
                tunnel: w1277 -> [w1294]
                tunnel: [w1293] -> w1276
                tunnel: w1275 -> [w1293]
                tunnel: [w1292] -> w1274
                tunnel: w1273 -> [w1292]
                tunnel: w1272 -> [w1291]
                tunnel: w1271 -> [w1290]
                tunnel: [w1283] -> w1269
                tunnel: w1268 -> [w1289]
                tunnel: w1267 -> [w1288]
                tunnel: w1266 -> [w1282]
                tunnel: w1265 -> [w1281]
                i -> [w1287]
                n424 = flat-sequence {
                  tunnel: w1291 -> [w1301]
                  tunnel: w1287 -> [w1299]
                  tunnel: w1289 -> [w1300]
                  tunnel: [w1299] -> w1286
                  tunnel: [w1298] -> w1284
                  tunnel: w1282 -> [w1297]
                  tunnel: w1290 -> [w1307]
                  tunnel: w1288 -> [w1306]
                  tunnel: w1286 -> [w1305]
                  tunnel: [w1304] -> w1285
                  tunnel: w1281 -> [w1303]
                  frame #0 {
                    n425 = call "DCIMG to TIFF conversion_multiple files.vi"("Volume number"=w1299, "IsSingleColor"=FALSE, "Input File Path"=w1301, "Input File Name"=w1297, "Output Path"=w1300) -> ("Error Out"=w1298:errorcluster)  [unwired: 5 in, 5 out]
                  }
                  frame #1 {
                    n426 = call "DCIMG to TIFF conversion_multiple files.vi"("Volume number"=w1305, "IsSingleColor"=FALSE, "Input File Path"=w1307, "Input File Name"=w1303, "Output Path"=w1306) -> ("Error Out"=w1304:errorcluster)  [unwired: 5 in, 5 out]
                  }
                }
                n427 = property on="Volume Indicator" class="Slide (strict)"("Value"=w1287) -> ()  [unwired: 2 in, 2 out]
                n428 = Merge Errors(w1285, w1284) -> (w1283:errorcluster)
              }
            }
          }
          n429 = local read "AutoFocus \n(move only piezo)"() -> (w1256:bool)
          n430 = local write "Acquisition status:"("Exporting DCIMG to TIFFs..." ("Program status")) -> ()
          n431 = case shown="True" w1256 {
            frame False {
            }
            frame True {
            }
          }
        }
        frame #3 {
          n432 = local write "Acquisition status:"("Done." ("Program status")) -> ()
          "File conversion Dual color" <- w1308
        }
      }
      n433 = Build Path(base path=w1138, name or relative path="Imaging  Conditions.txt") -> (appended path=w1139:path)
      n434 = call "MakeImagCondFileContents.vi"("Cluster"=w1135, "Position"=w1136, "StorageDirPath"=w1138) -> ("StringOutToFile"=w1137:string)  [unwired: 8 in]
      n435 = Write to Text File(file (use dialog)=w1139, text=w1137) -> (error out=w1134:errorcluster)  [unwired: 2 in, 2 out]
      n436 = call <userlib>:"tm_closecamera.vi"("error in (no error)"=w1162, "Handle in"=w1163) -> ("error out"=w1165:errorcluster)  [unwired: 9 in]
      n437 = call <userlib>:"tm_closecamera.vi"("error in (no error)"=w1161, "Handle in"=w1156) -> ("error out"=w1166:errorcluster)  [unwired: 9 in]
      n438 = Merge Errors(w1165, w1166) -> (w1164:errorcluster)
      n439 = call <userlib>:"tm_deinitialize.vi"("error in (no error)"=w1164) -> ("error out"=w1149:errorcluster)  [unwired: 10 in]
    }
  }
  "SPIMB DAQ Error" <- w81
  "SPIMA DAQ Error" <- w78
  "SPIM Camera Error" <- w70
  "Bottom Cam error" <- w50
  "Serial port errors" <- w49
  "Imag. cond. error out" <- w1
